vi "FingerMove.vi"() -> ()   [LabVIEW 2013]
uses:
  <vilib>/DAQmx/configure/timing.llb/DAQmx Timing (Implicit).vi
  <vilib>/DAQmx/create/channels.llb/DAQmx Create Channel (CO-Pulse Generation-Frequency).vi
  <vilib>/DAQmx/write.llb/DAQmx Write (Counter Frequency 1Chan 1Samp).vi
  <vilib>/DAQmx/write.llb/DAQmx Write (Digital 1D Bool NChan 1Samp 1Line).vi
  <vilib>/DAQmx/read.llb/DAQmx Read (Counter DBL 1Chan 1Samp).vi
  <vilib>/Platform/TimedLoop/XDataNode/wakeup.ctl
  <vilib>/Platform/TimedLoop/XDataNode/XDNodeRunTimeDep.lvlib
  <vilib>/Platform/TimedLoop/XDataNode/nitl_modes.ctl
  <vilib>/Platform/TimedLoop/XDataNode/timing_clust.ctl
  <vilib>/Platform/TimedLoop/XDataNode/XDataNode.xnode
  <vilib>/addons/Digital Filter Design/NI_DigFilterLicensed.lvlib
  <vilib>/addons/control/pid/NI_PID_pid.lvlib
  <vilib>/DAQmx/write.llb/DAQmx Write (Analog DBL 1Chan 1Samp).vi
  <vilib>/nisyscfg/nisyscfg.lvlib
  SubVIs/VariablesToString_Scalar.vi
  SubVIs/VariablesToString_Array.vi
  <vilib>/addons/control/pid/pid.llb/PID Advanced (DBL Array).vi
  <vilib>/addons/Digital Filter Design/Process.llb/DFD Filtering (PtByPt NChan).vi
  <vilib>/DAQmx/write.llb/DAQmx Write (Analog 1D DBL NChan 1Samp).vi
  SubVIs/VariablesToString_String.vi
  <vilib>/DAQmx/read.llb/DAQmx Read (Analog 1D DBL NChan 1Samp).vi
  <vilib>/addons/Digital Filter Design/_Objects.llb/DFD Filter Structure Type Selector.ctl
  <vilib>/addons/Digital Filter Design/_Objects.llb/DFD Filter Coef.ctl
  <vilib>/addons/Digital Filter Design/_Objects.llb/dfd_Internal Quantization Srcs.ctl
  <vilib>/addons/Digital Filter Design/_Objects.llb/dfd_Internal Quantization Settings.ctl
  <vilib>/addons/Digital Filter Design/_Objects.llb/DFD Coef Norm Type.ctl
  <vilib>/addons/Digital Filter Design/_Objects.llb/DFD Filter Obj.ctl
  <vilib>/Utility/miscctls.llb/LVBoundsTypeDef.ctl
  Control 1.ctl
panel:
  in  "Displacement":dbl[](array[numeric])=[4.95, 5.2, 3.9]
  in  "Middle Reverse Mode":bool
  out "Position, cm":T1(graph)
  out "#SuccessfulBlockTrials":u16
  out "IMT-%Correct":dbl
  out "IMT-Total":dbl
  out "IMT-Success":dbl
  out "MT-%Correct":dbl
  out "MT-Total":dbl
  out "MT-Success":dbl
  out "IT-%Correct":dbl
  out "IT-Total":dbl
  out "IT-Success":dbl
  out "IM-%Correct":dbl
  out "IM-Total":dbl
  out "IM-Success":dbl
  out "Thumb-%Correct":dbl
  out "Thumb-Total":dbl
  out "Thumb-Success":dbl
  out "Middle - %Correct":dbl
  out "Middle - Total":dbl
  out "Middle-Success":dbl
  out "Index-%Correct":dbl
  out "Index-Total":dbl
  out "Index-Success":dbl
  in  "Vis_Center_Y":dbl=0.6
  in  "Vis_Center X":dbl=0.6
  out "#TotalBlockTrials":u16
  in  "Rand_BlockSize":u16=5
  in  "Monkey":string(combo)="Izzle"
  out "GetHostTimeVI":path=path "E:/Code/Tasks/SubVIs/GetHostTime.vi"
  out "AutoCentraVI":path=path "E:/Code/Tasks/SubVIs/AutoCentral.vi"
  out "TaskFolder":path=path "E:/Code/Tasks/FingerMove"
  out "Recording?":bool
  out "CerebusFolder":string="20130418-111956"
  out "StopRecording":bool
  out "Scalefactor":dbl=0.3
  in  "Blank 2":picture
  out "DrawSize 2":T2={"Width"=499, "Height"=304}
  out "Display 2":picture
  out "FingerNum":dbl=1.0
  out "AbortTrials":dbl caption="Total # of Aborts"
  out "FailureTrials":dbl caption="Total # of Failures"
  in  "TrainThresh":dbl[](array[numeric])=[0.5, 0.5, 0.5]
  out "Status":enum16{"In", "Out"}(ring)=enum."Out"
  in  "Radius":dbl=0.44 caption="SuccessRadius"
  in  "MultR":dbl=250.0 caption="DisplayRad"
  out "DrawSize":T2={"Width"=1662, "Height"=1015}
  out "PercentCorrect":dbl caption="Overall - %Correct" format="%#_4g"
  out "SuccessfulTrials":dbl caption="Overall - Successful"
  in  "Pause":bool
  in  "Finger":T3={"Index"=TRUE, "Middle"=FALSE, "Thumb"=FALSE}
  in  "TargetPos":dbl[](array[numeric])=[4.95, 5.2, 3.9]
  in  "Blank":picture
  in  "PIDLimit":dbl=0.5 caption="MaxDutyCycle" min=0.0 max=1.0 step=0.01 format="%.2f"
  out "LP_LoadCell":T4={"mSRate_Fs"=500.0, "mSRate_Version"="2.0", "mSRate_Comments"="", "mSRate_OrgCoef"={"type"=enum."IIR Cascaded Second Order Sections Form II Transposed", "gain"=1.0, "coef a (k)"=[-0.36952737735124136, 0.1958157126558331], "coef b (v)"=[0.20657208382614795, 0.4131441676522959, 0.20657208382614795]}, "mSRate_CurCoef"={"type"=enum."IIR Cascaded Second Order Sections Form II Transposed", "gain"=1.0, "coef a (k)"=[-0.36952737735124136, 0.1958157126558331], "coef b (v)"=[0.20657208382614795, 0.4131441676522959, 0.20657208382614795]}, "mSRate_Quantized?"=FALSE, "mSRate_QCoef"={"type"=enum."Undefined", "gain"=1.0, "coef a (k)"=[], "coef b (v)"=[]}, "mSRate_QSettings"=[], "mSRate_Order"=2, "mSRate_Scaling"={"mSRate_ScaleByPowerOf2?"=FALSE, "mSRate_ScaleType"=enum."No Norm"}} {"mSRate_QSettings"."source" items=["Coef a/k"=0, "Coef b/v"=7, "Input"=1, "Output"=2, "Multiplicand"=3, "Product"=4, "Sum"=5, "Delay"=6, "Gain"=8]}
  out "PWMTaskA":refnum<k21>
  out "PIDSlowLoop":bool
  out "PIDLoopTime(us)":i64=881 caption="Actual Loop Period (us)"
  out "PIDLoopPeriod(s)":dbl=0.002 caption="Loop Period PID (s)" format="%#_10g"
  out "PWMTaskB":refnum<k21>
  in  "Stop":bool
  out "SetPoint":dbl[](array[numeric])=[1.0, 2.0, 1.0] caption="Set Point" min=-10.0 max=10.0 step=1.0
  in  "PIDLoopFreq(Hz)":dbl=500.0 caption="Loop Period (us)"
  out "PWMTaskC":refnum<k21>
  out "MotorDir":bool[](array[boolean])=[TRUE, TRUE, TRUE]
  in  "LP_LoadCell(Hz)":dbl=100.0
  in  "BndrsCluster":T10={"InwardLimit(%)"=[0.75, 0.8, 0.6], "OutwardLimit(%)"=[0.25, 0.2, 0.4], "SpringCnst"=[5.0, 5.0, 5.0]} caption="Boundaries"
  out "EncMax":dbl[](array[numeric])
  in  "PWMFreq(Hz)":dbl=20000.0 caption="PWM (Hz)" format="%#.6f"
  in  "PIDGains":T11={"proportional high (Kc)"=0.2, "integral high (Ti, min)"=0.0, "derivative high (Td, min)"=0.0, "derivative low (Td, min)"=0.0, "integral low (Ti, min)"=0.0, "proportional low (Kc)"=0.1} caption="PID Gains"
  out "PIDGainsOut":T12(array[cluster])=[{"proportional gain (Kc)"=0.4600000000000001, "integral time (Ti, min)"=0.0, "derivative time (Td, min)"=0.0}, {"proportional gain (Kc)"=0.42000000000000004, "integral time (Ti, min)"=0.0, "derivative time (Td, min)"=0.0}, {"proportional gain (Kc)"=0.4600000000000001, "integral time (Ti, min)"=0.0, "derivative time (Td, min)"=0.0}]
  in  "Linearity":dbl=1.0 format="%.2f"
  out "Outcome":string="--"
  out "Current State":T13(ring)=enum."Acquire Start"
  out "Finalize":enum16{"Reward", "Cerebus", "Reset"}(ring)
  out "LoopCount":u64=13080
  out "TrialCount":i32=1 caption="Overall - Total Trials"
  out "EncPos":cluster{"[0]":dbl, "[1]":dbl, "[2]":dbl}(graph) caption="Position"
  in  "InitialPos":dbl[](array[numeric])=[4.95, 5.2, 3.9]
  out "LoadCell":cluster{"[0]":dbl, "[1]":dbl, "[2]":dbl}(graph)={"[0]"=0.5361853302770733, "[1]"=0.5356007172382269, "[2]"=0.5346289515190896} caption="Force, lbs"
  out "SetPtOut":cluster{"[0]":dbl, "[1]":dbl, "[2]":dbl}(graph)={"[0]"=1.0, "[1]"=2.0, "[2]"=1.0} caption="Set Point, lbs"
  in  "InitialForce":dbl[](array[numeric])=[1.0, 2.0, 1.0] min=-10.0 max=10.0 step=1.0
  in  "RandFinger":bool
  out "StartTime":timestamp=timestamp(3449121258.124381 s since 1904-01-01)
  out "TaskType":string="FingerMove.vi"
  out "DatabaseUDL":path=path "E:/Data/Setup2Database.udl"
  in  "RecordsSelection":string(combo)
  in  "Database":T14={"ExperimentDate"=timestamp(3449121258.124381 s since 1904-01-01), "ImplantDate"=timestamp(3449023200 s since 1904-01-01), "CerebusFolder"="20130418-111956", "Experimenter"="Cody Barton", "NHPName"="Frak", "DeviceType"="USEA", "DeviceSerial"="CG-64BPX-F419", "DeviceHemisphere"="right", "DeviceRegion"="median nerve", "TaskType"="FingerMove.vi", "TaskComments"="test123", "RecordingComments"="test123", "GeneralObservations"="test123"}
  in  "CerebusConfigFile":path=path "E:/Code/Tasks/FingerMove/CerebusConfigBehavior20130507.mat"
  in  "Timing":T15={"JuiceTime"=1700.0, "AbortTime"=2000.0, "ARD"=1500.0, "HoldTime"=500.0, "ASD"=1000.0}
  out "Display":picture
  out "LoopPeriod":u64=10
  out "SlowLoop":bool
  out "LoopTime":i64=381
  # "Do not place ';' or '=' in the comment fields"
  # "all time in ms"
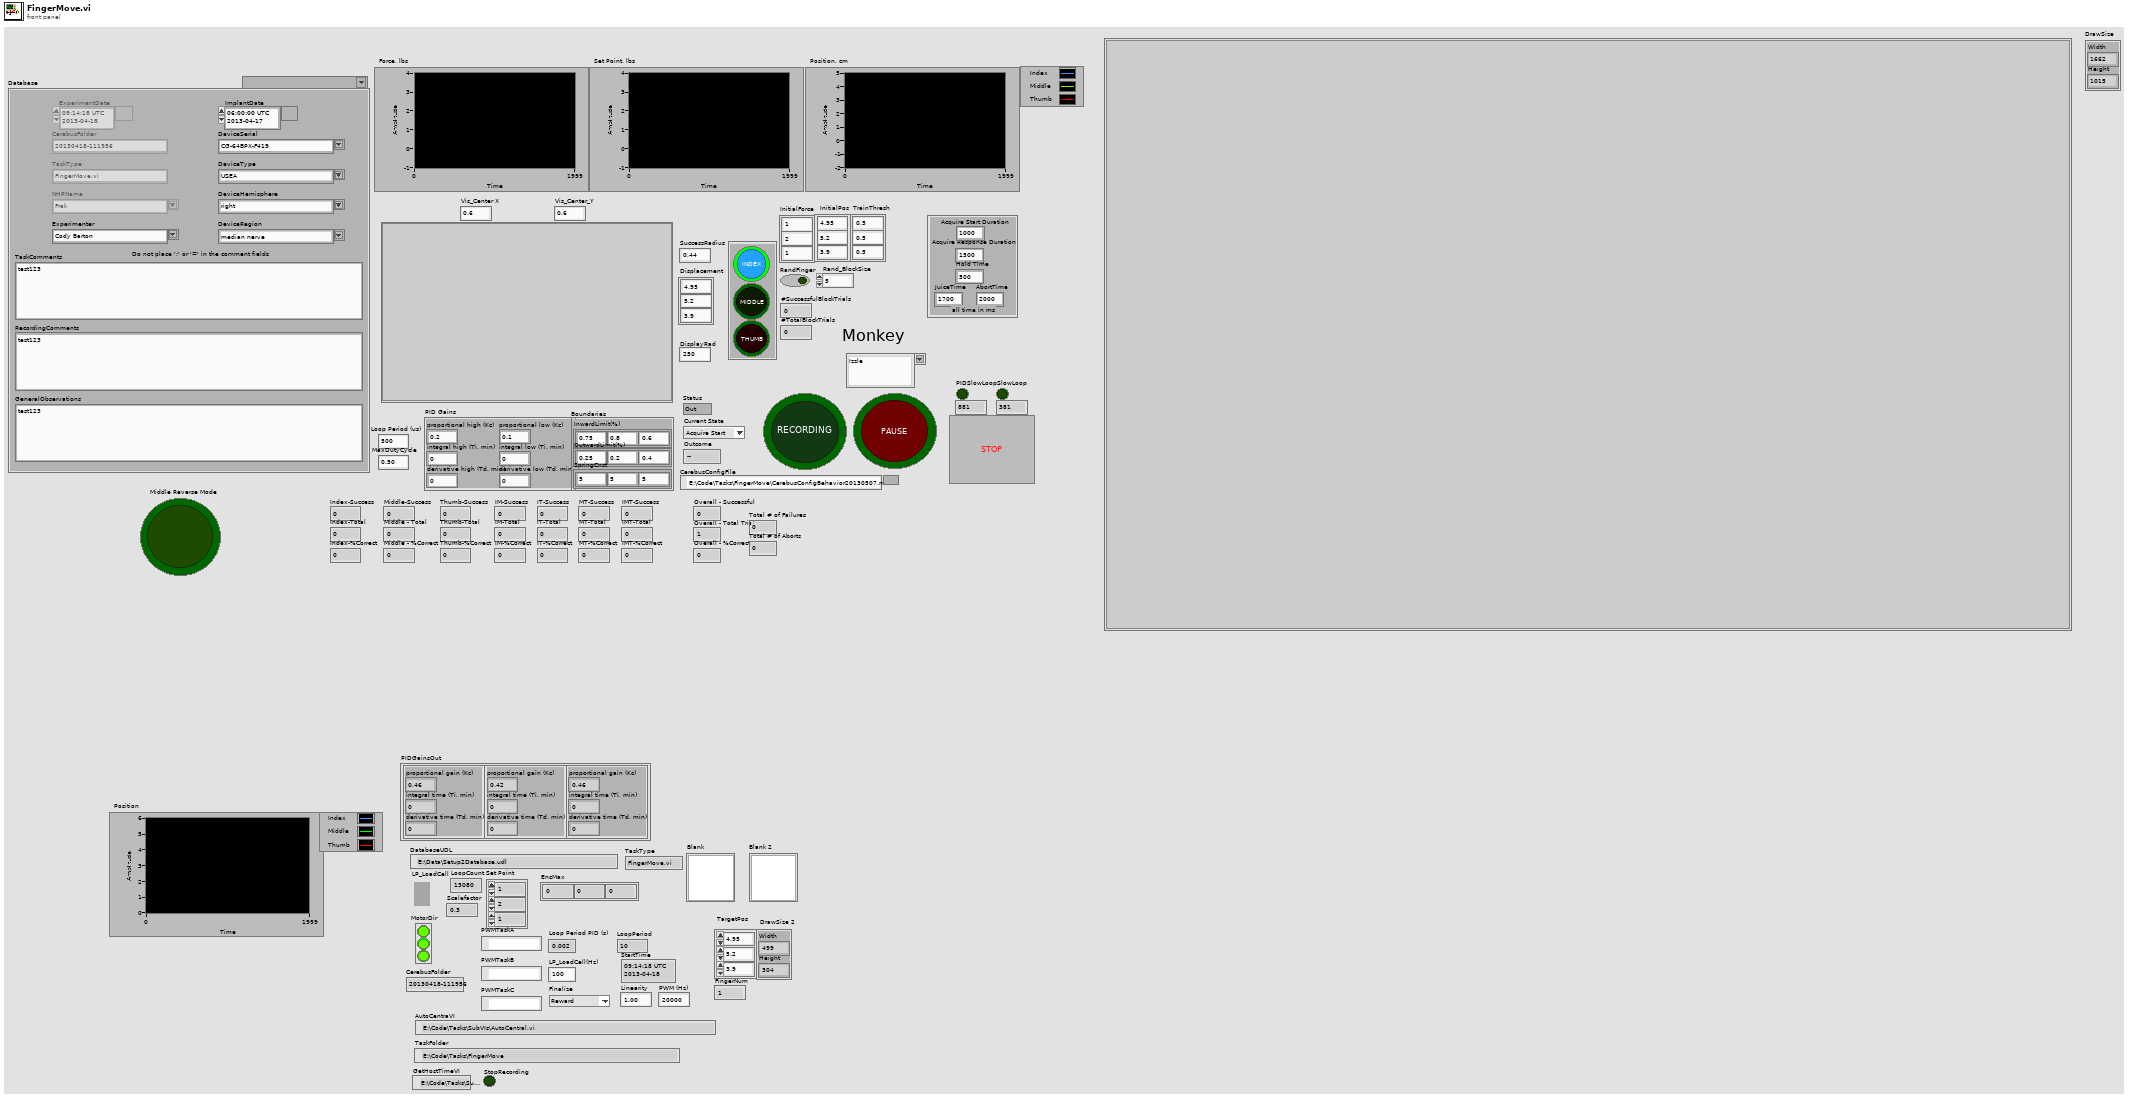
[diagram p1: front panel]
types:
  T1 = cluster{"[0]":dbl, "[1]":dbl, "[2]":dbl, "[3]":dbl, "[4]":dbl, "[5]":dbl, "[6]":dbl, "[7]":dbl, "[8]":dbl}
  T2 = typedef "LVBoundsTypeDef.ctl" = cluster{"Width":u32, "Height":u32}
  T3 = cluster{"Index":bool, "Middle":bool, "Thumb":bool}
  T4 = typedef "NI_DigFilterLicensed.lvlib/DFD Filter Obj.ctl" = cluster{"mSRate_Fs":dbl, "mSRate_Version":string, "mSRate_Comments":string, "mSRate_OrgCoef":T5, "mSRate_CurCoef":T5, "mSRate_Quantized?":bool, "mSRate_QCoef":T5, "mSRate_QSettings":T7[], "mSRate_Order":i32, "mSRate_Scaling":cluster{"mSRate_ScaleByPowerOf2?":bool, "mSRate_ScaleType":T9}}
  T5 = typedef "NI_DigFilterLicensed.lvlib/DFD Filter Coef.ctl" = cluster{"type":T6, "gain":dbl, "coef a (k)":dbl[], "coef b (v)":dbl[]}
  T6 = typedef "NI_DigFilterLicensed.lvlib/DFD Filter Structure Type Selector.ctl" = enum16{"Undefined", "FIR Direct Form", "FIR Direct Form Transposed", "FIR Symmetric", "FIR Antisymmetric", "IIR Direct Form I", "IIR Direct Form I Transposed", "IIR Direct Form II", "IIR Direct Form II Transposed", "IIR Cascaded Second Order Sections Form I", "IIR Cascaded Second Order Sections Form I Transposed", "IIR Cascaded Second Order Sections Form II", "IIR Cascaded Second Order Sections Form II Transposed", "Lattice Allpass (basic sections)", "Lattice Allpass (one multiplier sections)", "Lattice Allpass (normalized sections)", "Lattice AR (basic sections)", "Lattice AR (one multiplier sections)", "Lattice AR (normalized sections)", "Lattice MA (minimum phase)", "Lattice MA (maximum phase)", "Lattice ARMA (basic sections)", "Lattice ARMA (one multiplier sections)", "Lattice ARMA (normalized sections)"}
  T7 = typedef "NI_DigFilterLicensed.lvlib/dfd_Internal Quantization Settings.ctl" = cluster{"source":T8, "wl":i16, "iwl":i16, "overflow mode":enum16{"Saturation", "Wrap"}, "rounding mode":enum16{"Nearest", "Truncation"}, "signed?":bool}
  T8 = typedef "NI_DigFilterLicensed.lvlib/dfd_Internal Quantization Srcs.ctl" = u16
  T9 = typedef "NI_DigFilterLicensed.lvlib/DFD Coef Norm Type.ctl" = enum16{"No Norm", "Time Domain 1-Norm", "Time Domain 2-Norm", "Time Domain Inf-Norm"}
  T10 = cluster{"InwardLimit(%)":dbl[], "OutwardLimit(%)":dbl[], "SpringCnst":dbl[]}
  T11 = cluster{"proportional high (Kc)":dbl, "integral high (Ti, min)":dbl, "derivative high (Td, min)":dbl, "derivative low (Td, min)":dbl, "integral low (Ti, min)":dbl, "proportional low (Kc)":dbl}
  T12 = cluster{"proportional gain (Kc)":dbl, "integral time (Ti, min)":dbl, "derivative time (Td, min)":dbl}[]
  T13 = enum16{"Initialize", "Acquire Start", "Acquire Response", "Finalize"}
  T14 = cluster{"ExperimentDate":timestamp, "ImplantDate":timestamp, "CerebusFolder":string, "Experimenter":string, "NHPName":string, "DeviceType":string, "DeviceSerial":string, "DeviceHemisphere":string, "DeviceRegion":string, "TaskType":string, "TaskComments":string, "RecordingComments":string, "GeneralObservations":string}
  T15 = typedef "Control 1.ctl" = cluster{"JuiceTime":dbl, "AbortTime":dbl, "ARD":dbl, "HoldTime":dbl, "ASD":dbl}
  T16 = enum16{"Initialize", "String", "Start", "New Session", "Stop", "Resume", "Close"}
  T17 = cluster{"JuiceTime":dbl, "AbortTime":dbl, "ARD":dbl, "HoldTime":dbl, "ASD":dbl}
  T18 = cluster{"ExperimentDate":timestamp, "ImplantDate":timestamp, "CerebusFolder":string, "Experimenter":string, "NHP Name":string, "DeviceType":string, "DeviceSerial":string, "DeviceHemisphere":string, "DeviceRegion":string, "TaskType":string, "TaskComments":string, "RecordingComments":string, "GeneralObservations":string}
  T19 = enum16{"SaveConfiguration", "StartRecording", "StopRecording"}
  T20 = typedef "XDNodeRunTimeDep.lvlib/timing_clust.ctl" = cluster{"Expected End [f-1]":u64, "Actual End [f-1]":u64, "Finished Late? [f-1]":bool, "Expected End [i-1]":u64, "Actual End [i-1]":u64, "Finished Late? [i-1]":bool, "Expected Start [i]":u64, "Actual Start [i]":u64, "Expected Start [f]":u64, "Actual Start [f]":u64, "Source Name":string, "Structure Name":string, "Period":i64, "Deadline":i64, "Offset":i64, "Start":i64, "Priority":i32, "Timeout":i32, "Mode":T21, "Wakeup Reason":T22, "Error":errorcluster, "Source Type":string, "Secondary Source Type":string, "Global End Time":u64, "Global Start Time":u64, "Frame Duration":u64, "Iteration Duration":u64, "Assigned CPU":i32, "I/O Scan Engine Mode":u32}
  T21 = typedef "XDNodeRunTimeDep.lvlib/nitl_modes.ctl" = enum32{"No Change", "Process missed periods, maintain original phase", "Discard missed periods, maintain original phase", "Process missed periods, ignore original phase", "Discard missed periods, ignore original phase"}
  T22 = typedef "XDNodeRunTimeDep.lvlib/wakeup.ctl" = enum32{"Normal", "Aborted", "Asynchronous wakeup", "Timing source error", "Timed loop error", "Timeout"}
  T23 = enum16{"Lowpass", "Highpass", "Bandpass", "Bandstop"}
  T24 = cluster{"left":i16, "left":i16, "Width":u32, "Height":u32}
  T25 = cluster{"SetPointOut[0]":dbl, "SetPointOut[1]":dbl, "SetPointOut[2]":dbl}
  T26 = cluster{"signal out[0]":dbl, "signal out[1]":dbl, "signal out[2]":dbl}
  T27 = typedef "LVAllMonitorsDisplayTypeDef.ctl" = cluster{"Bounds":cluster{"Left":i16, "Top":i16, "Right":i16, "Bottom":i16}, "Depth":i16}[]
  T28 = cluster{"Disp.AllMonitors[0]":cluster{"Bounds":cluster{"Left":i16, "Top":i16, "Right":i16, "Bottom":i16}, "Depth":i16}, "Disp.AllMonitors[1]":cluster{"Bounds":cluster{"Left":i16, "Top":i16, "Right":i16, "Bottom":i16}, "Depth":i16}, "Disp.AllMonitors[2]":cluster{"Bounds":cluster{"Left":i16, "Top":i16, "Right":i16, "Bottom":i16}, "Depth":i16}, "Disp.AllMonitors[3]":cluster{"Bounds":cluster{"Left":i16, "Top":i16, "Right":i16, "Bottom":i16}, "Depth":i16}, "Disp.AllMonitors[4]":cluster{"Bounds":cluster{"Left":i16, "Top":i16, "Right":i16, "Bottom":i16}, "Depth":i16}, "Disp.AllMonitors[5]":cluster{"Bounds":cluster{"Left":i16, "Top":i16, "Right":i16, "Bottom":i16}, "Depth":i16}, "Disp.AllMonitors[6]":cluster{"Bounds":cluster{"Left":i16, "Top":i16, "Right":i16, "Bottom":i16}, "Depth":i16}, "Disp.AllMonitors[7]":cluster{"Bounds":cluster{"Left":i16, "Top":i16, "Right":i16, "Bottom":i16}, "Depth":i16}, "Disp.AllMonitors[8]":cluster{"Bounds":cluster{"Left":i16, "Top":i16, "Right":i16, "Bottom":i16}, "Depth":i16}}
  T29 = typedef "LVRectTypeDef.ctl" = cluster{"Left":i16, "Top":i16, "Right":i16, "Bottom":i16}
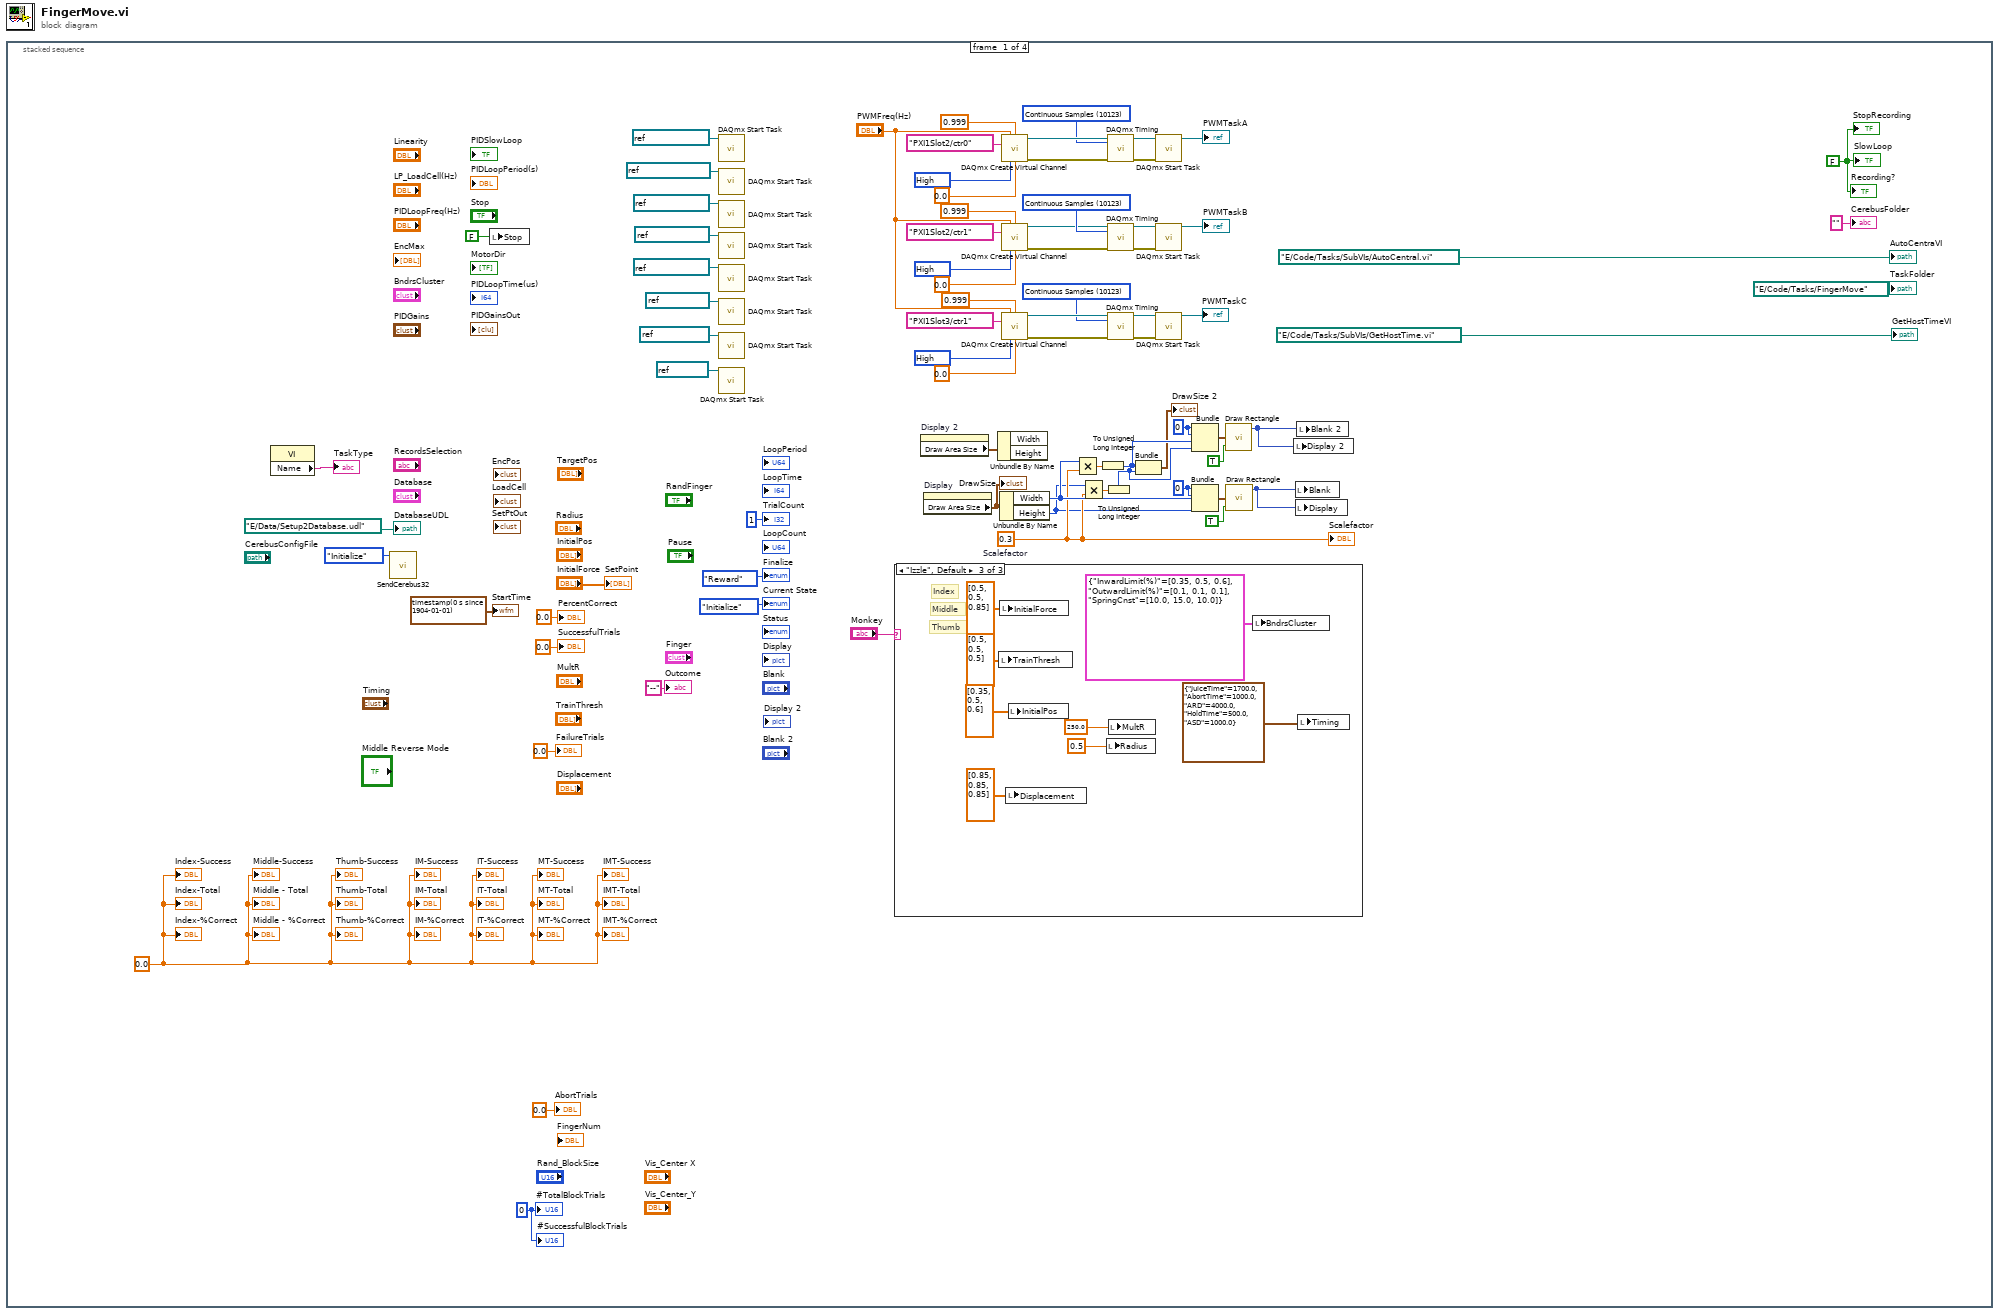
[diagram p0: block diagram]
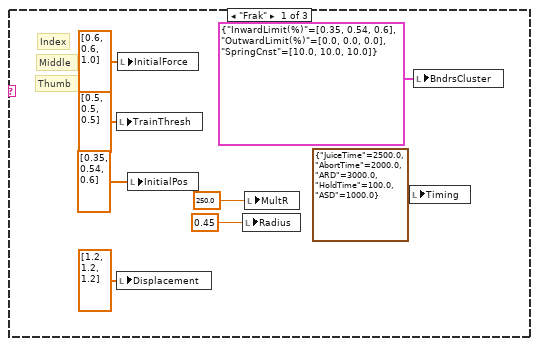
[diagram p2: hidden frame]
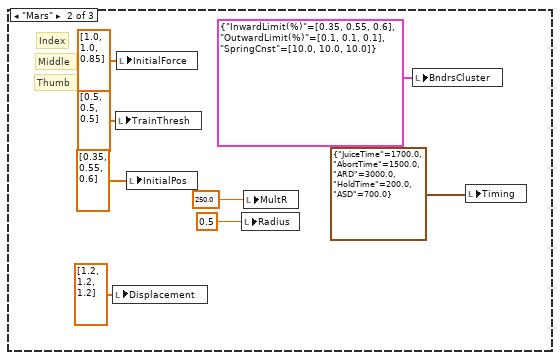
[diagram p3: hidden frame]
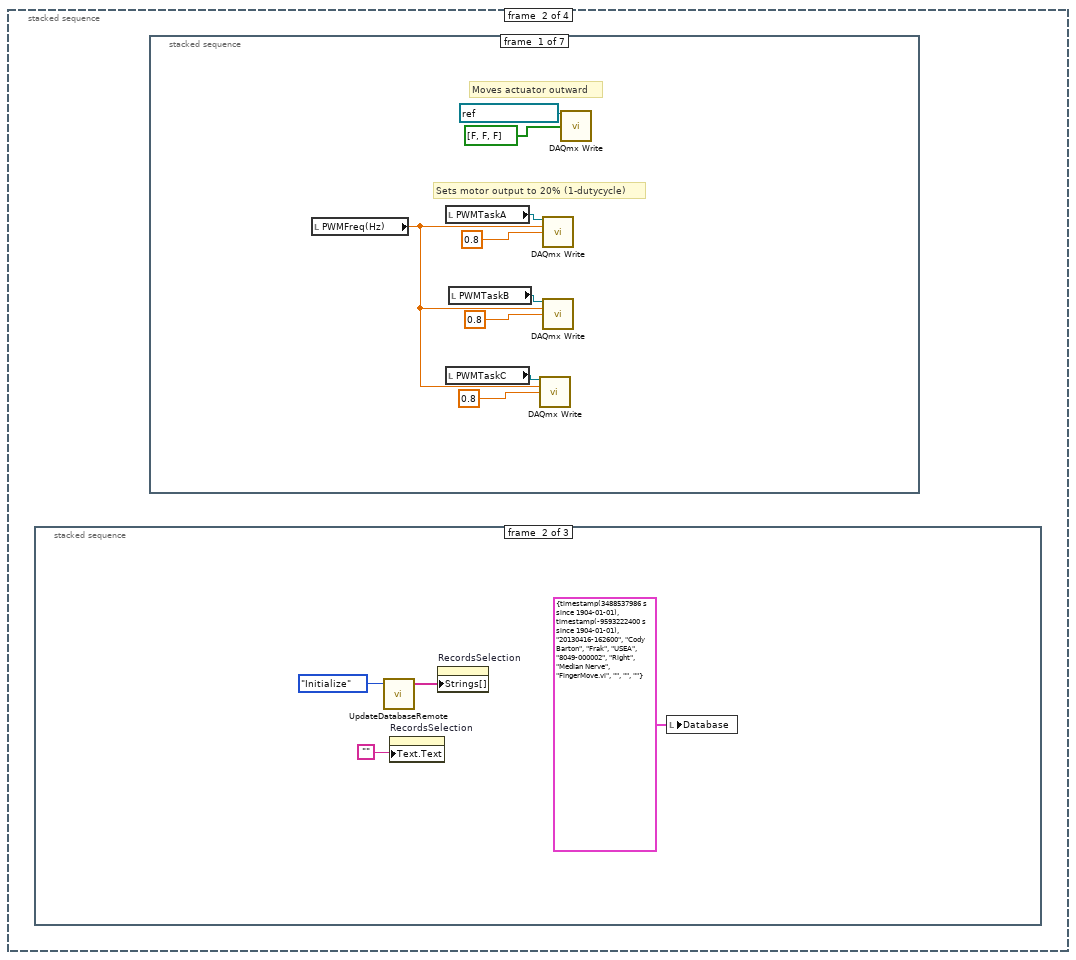
[diagram p4: hidden frame]
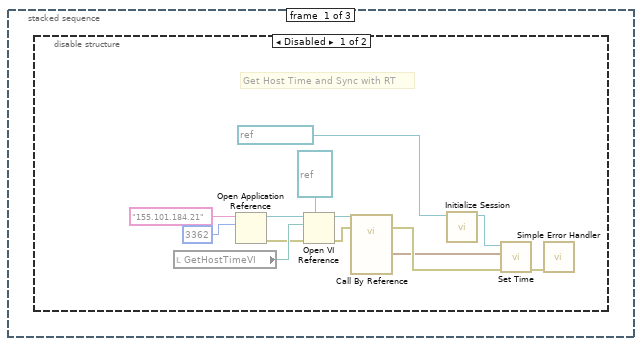
[diagram p5: hidden frame]
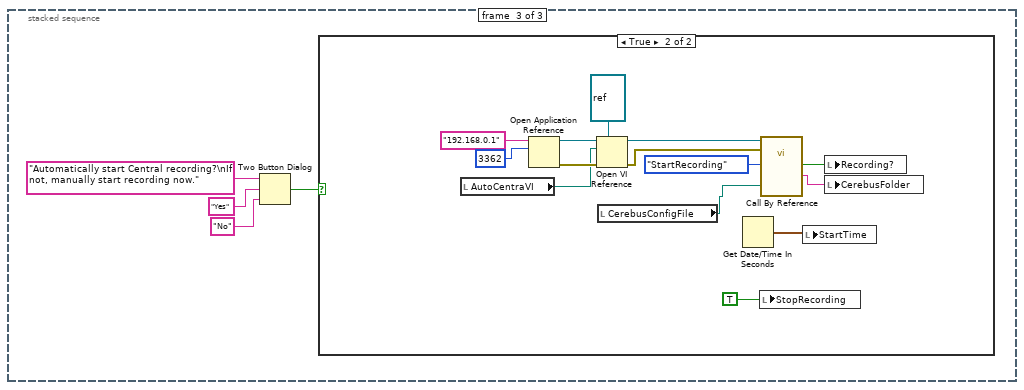
[diagram p7: hidden frame]
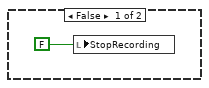
[diagram p8: hidden frame]
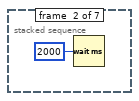
[diagram p9: hidden frame]
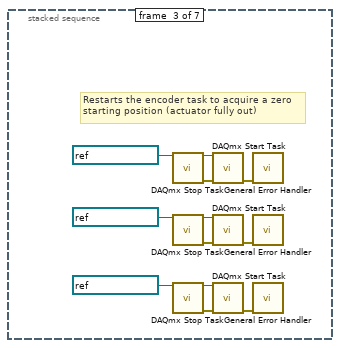
[diagram p10: hidden frame]
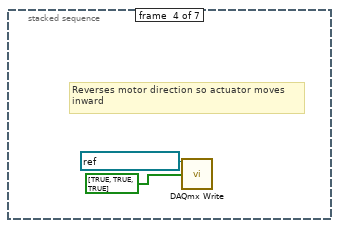
[diagram p11: hidden frame]
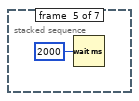
[diagram p12: hidden frame]
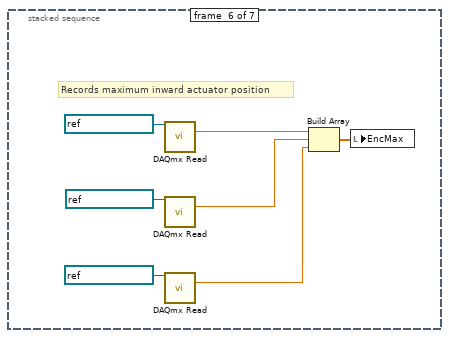
[diagram p13: hidden frame]
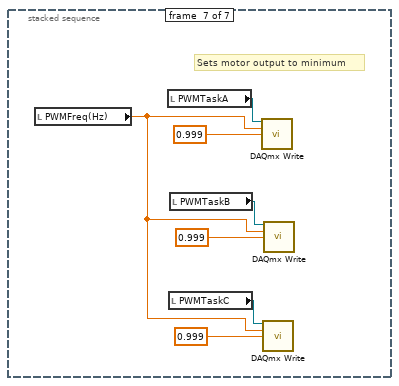
[diagram p14: hidden frame]
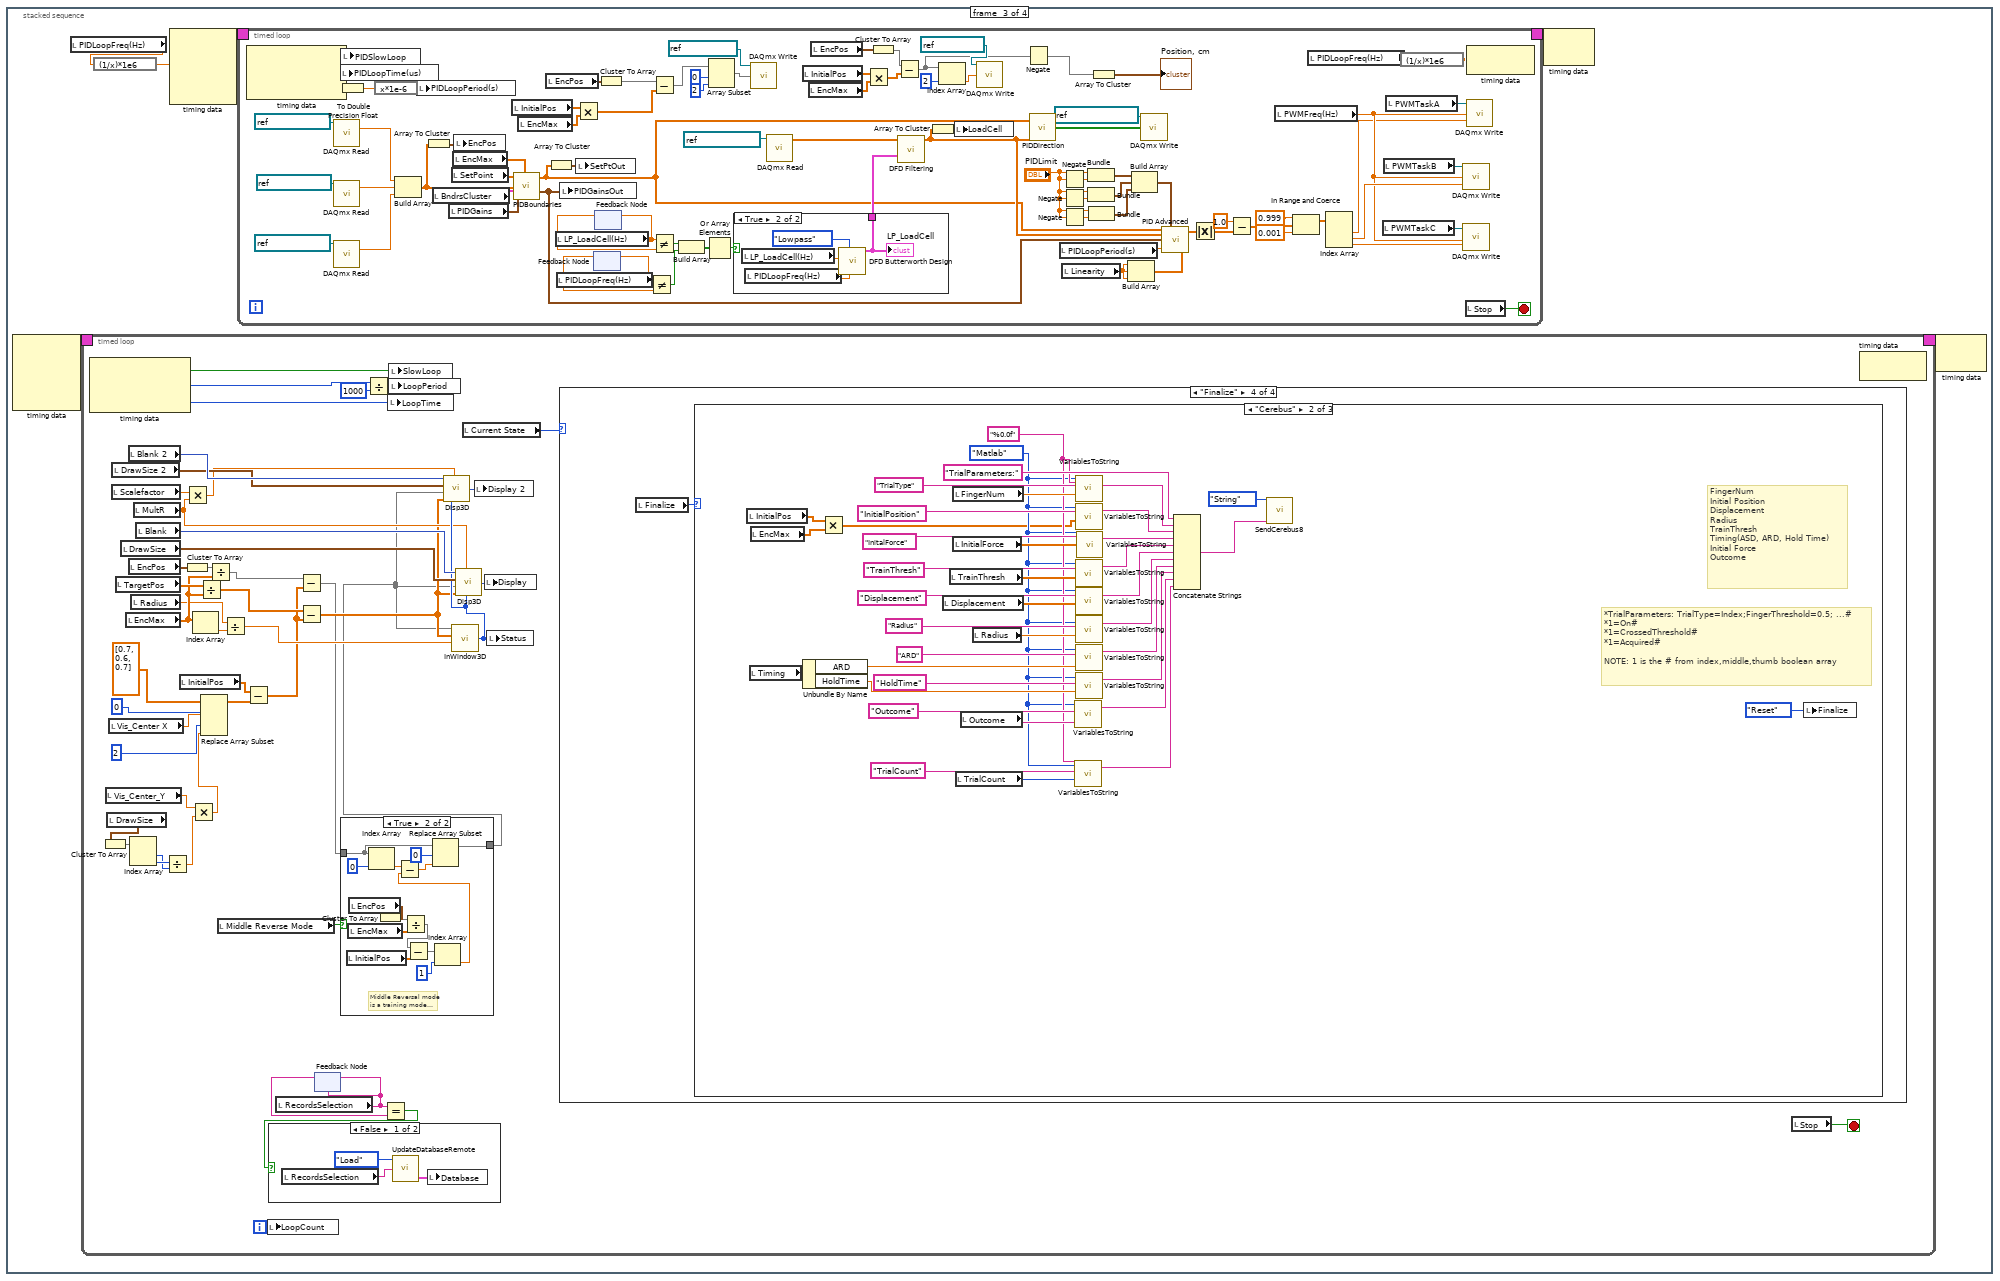
[diagram p15: hidden frame]
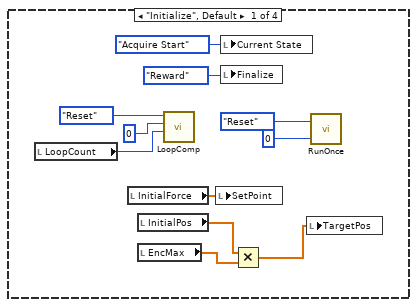
[diagram p18: hidden frame]
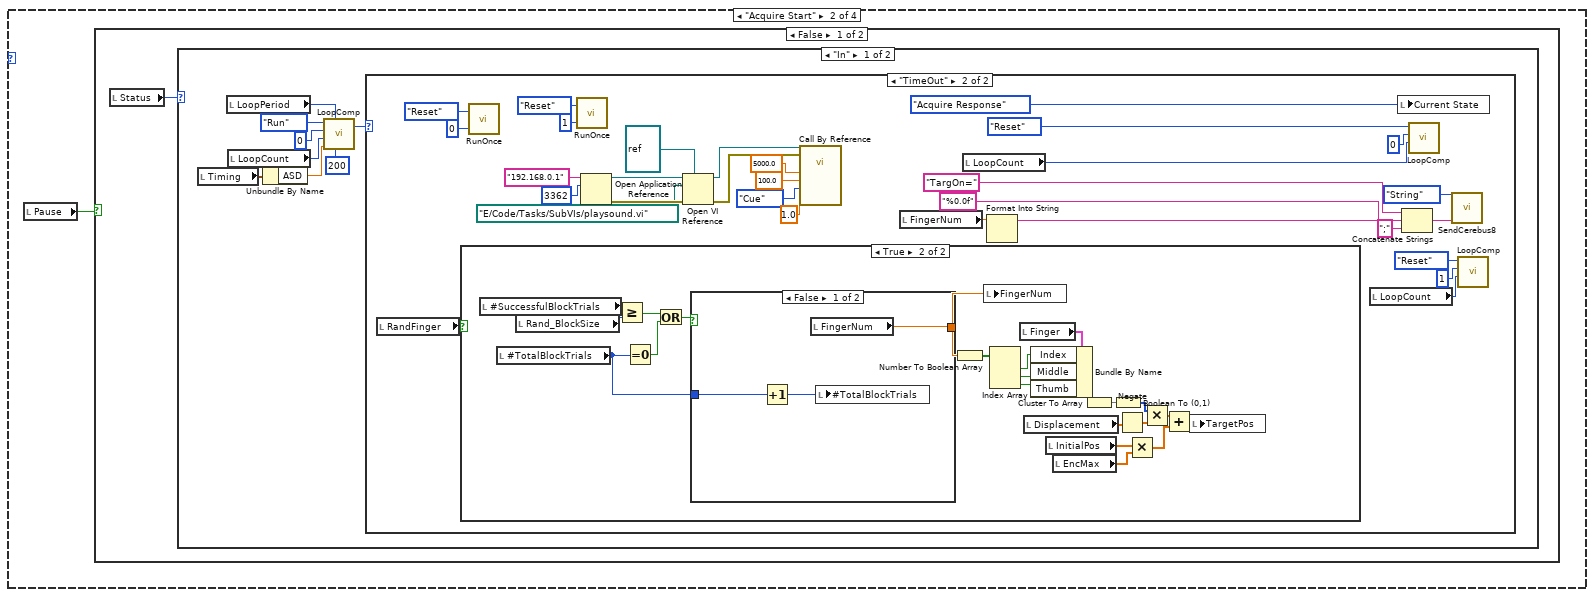
[diagram p19: hidden frame]
diagram:
  n1 = stacked-sequence {
    frame #0 {
      w2 = 0.0
      w1 = 0
      w3 = FALSE ("StopRecording")
      w21 = 0.3  # Scalefactor
      w25 = i16 0 ("left")
      w29 = i16 0 ("left")
      w52 = 10192 items=["High"=10192, "Low"=10214] ("idle state")
      w46 = 10123 items=["Finite Samples"=10178, "Continuous Samples"=10123] ("sample mode")
      w59 = 10192 items=["High"=10192, "Low"=10214] ("idle state")
      w65 = 10123 items=["Finite Samples"=10178, "Continuous Samples"=10123] ("sample mode")
      w76 = 10192 items=["High"=10192, "Low"=10214] ("idle state")
      w69 = 10123 items=["Finite Samples"=10178, "Continuous Samples"=10123] ("sample mode")
      n2 = property class="VI"() -> ("Name"=→"TaskType":string)  [unwired: 2 in, 2 out]
      n3 = call "SendCerebus32.vi"("Mode"=T16."Initialize") -> ()  [unwired: 4 in]
      n4 = local write "Stop"(FALSE ("stop")) -> ()
      n5 = call <vilib>:"DAQmx Start Task.vi"("task/channels in"=refnum<k21> "ForceInABC") -> ()  [unwired: 13 in, 2 out]
      n6 = call <vilib>:"DAQmx Start Task.vi"("task/channels in"=refnum<k21> "MotorDirABC") -> ()  [unwired: 13 in, 2 out]
      n7 = call <vilib>:"DAQmx Start Task.vi"("task/channels in"=refnum<k21> "PositionInA") -> ()  [unwired: 13 in, 2 out]
      n8 = call <vilib>:"DAQmx Start Task.vi"("task/channels in"=refnum<k21> "PositionInB" ("task")) -> ()  [unwired: 13 in, 2 out]
      n9 = call <vilib>:"DAQmx Start Task.vi"("task/channels in"=refnum<k21> "PositionInC") -> ()  [unwired: 13 in, 2 out]
      n10 = call <vilib>:"DAQmx Start Task.vi"("task/channels in"=refnum<k21> "PosOutT" ("task")) -> ()  [unwired: 13 in, 2 out]
      n11 = call <vilib>:"DAQmx Start Task.vi"("task/channels in"=refnum<k21> "PosOutIM") -> ()  [unwired: 13 in, 2 out]
      n12 = call <vilib>:"DAQmx Start Task.vi"("task/channels in"=refnum<k21> "sound") -> ()  [unwired: 13 in, 2 out]
      n13 = case shown="\"Izzle\", Default" "Monkey" {
        frame "Frak" {
          # "Thumb"
          # "Middle"
          # "Index"
          n14 = local write "TrainThresh"(dbl[] [0.5, 0.5, 0.5] ("InitialForce")) -> ()
          n15 = local write "Displacement"(dbl[] [1.2, 1.2, 1.2] ("InitialPos")) -> ()
          n16 = local write "InitialForce"(dbl[] [0.6, 0.6, 1.0] ("InitialForce")) -> ()
          n17 = local write "InitialPos"(dbl[] [0.35, 0.54, 0.6] ("InitialPos")) -> ()
          n18 = local write "Radius"(0.45 ("Displacement")) -> ()
          n19 = local write "MultR"(250.0 ("Displacement")) -> ()
          n20 = local write "Timing"(T17 {"JuiceTime"=2500.0, "AbortTime"=2000.0, "ARD"=3000.0, "HoldTime"=100.0, "ASD"=1000.0} ("Timing")) -> ()
          n21 = local write "BndrsCluster"(T10 {"InwardLimit(%)"=[0.35, 0.54, 0.6], "OutwardLimit(%)"=[0.0, 0.0, 0.0], "SpringCnst"=[10.0, 10.0, 10.0]} ("BndrsCluster")) -> ()
        }
        frame "Mars" {
          # "Thumb"
          # "Middle"
          # "Index"
          n22 = local write "Displacement"(dbl[] [1.2, 1.2, 1.2] ("InitialPos")) -> ()
          n23 = local write "TrainThresh"(dbl[] [0.5, 0.5, 0.5] ("InitialForce")) -> ()
          n24 = local write "InitialForce"(dbl[] [1.0, 1.0, 0.85] ("InitialForce")) -> ()
          n25 = local write "InitialPos"(dbl[] [0.35, 0.55, 0.6] ("InitialPos")) -> ()
          n26 = local write "Radius"(0.5 ("Displacement")) -> ()
          n27 = local write "MultR"(250.0 ("Displacement")) -> ()
          n28 = local write "BndrsCluster"(T10 {"InwardLimit(%)"=[0.35, 0.55, 0.6], "OutwardLimit(%)"=[0.1, 0.1, 0.1], "SpringCnst"=[10.0, 10.0, 10.0]} ("BndrsCluster")) -> ()
          n29 = local write "Timing"(T17 {"JuiceTime"=1700.0, "AbortTime"=1500.0, "ARD"=3000.0, "HoldTime"=200.0, "ASD"=700.0} ("Timing")) -> ()
        }
        frame "Izzle", Default {
          # "Thumb"
          # "Middle"
          # "Index"
          n30 = local write "TrainThresh"(dbl[] [0.5, 0.5, 0.5] ("InitialForce")) -> ()
          n31 = local write "InitialForce"(dbl[] [0.5, 0.5, 0.85] ("InitialForce")) -> ()
          n32 = local write "Displacement"(dbl[] [0.85, 0.85, 0.85] ("InitialForce")) -> ()
          n33 = local write "InitialPos"(dbl[] [0.35, 0.5, 0.6] ("InitialPos")) -> ()
          n34 = local write "Radius"(0.5 ("Displacement")) -> ()
          n35 = local write "MultR"(250.0 ("Displacement")) -> ()
          n36 = local write "BndrsCluster"(T10 {"InwardLimit(%)"=[0.35, 0.5, 0.6], "OutwardLimit(%)"=[0.1, 0.1, 0.1], "SpringCnst"=[10.0, 15.0, 10.0]} ("BndrsCluster")) -> ()
          n37 = local write "Timing"(T17 {"JuiceTime"=1700.0, "AbortTime"=1000.0, "ARD"=4000.0, "HoldTime"=500.0, "ASD"=1000.0} ("Timing")) -> ()
        }
      }
      n38 = property on="Display 2" class="Pict"() -> ("Draw Area Size"=w24:T2)  [unwired: 2 in, 2 out]
      n39 = property on="Display" class="Pict"() -> ("Draw Area Size"=w28:T2)  [unwired: 2 in, 2 out]
      "DrawSize" <- w28
      n40 = Unbundle By Name(w24) -> ()  [unwired: 2 out]
      n41 = Unbundle By Name(w28) -> ("Width"=w23:u32, "Height"=w20:u32)
      n42 = call-poly <vilib>:"DAQmx Create Virtual Channel.vi"("frequency"="PWMFreq(Hz)", "duty cycle"=0.999, "counter"=tag "PXI1Slot2/ctr0", "idle state"=w76, "initial delay"=0.0) -> ("task out"=w72:refnum<k21>, "error out"=w73:errorcluster)  [unwired: 9 in]
      n43 = call-poly <vilib>:"DAQmx Create Virtual Channel.vi"("frequency"="PWMFreq(Hz)", "duty cycle"=0.999, "counter"=tag "PXI1Slot2/ctr1", "idle state"=w59, "initial delay"=0.0) -> ("task out"=w62:refnum<k21>, "error out"=w61:errorcluster)  [unwired: 9 in]
      n44 = call-poly <vilib>:"DAQmx Create Virtual Channel.vi"("frequency"="PWMFreq(Hz)", "duty cycle"=0.999, "counter"=tag "PXI1Slot3/ctr1", "idle state"=w52, "initial delay"=0.0) -> ("task out"=w49:refnum<k21>, "error out"=w50:errorcluster)  [unwired: 9 in]
      n45 = Multiply(x=w23, y=w21) -> (x*y=w22:dbl)
      n46 = Multiply(x=w20, y=w21) -> (x*y=w19:dbl)
      n47 = To Unsigned Long Integer(number=w22) -> (unsigned 32bit integer=w18:u32)
      n48 = To Unsigned Long Integer(number=w19) -> (unsigned 32bit integer=w17:u32)
      n49 = call-poly <vilib>:"DAQmx Timing.vi"("task/channels in"=w72, "sample mode"=w69, "error in"=w73) -> ("task out"=w70:refnum<k21>, "error out"=w71:errorcluster)  [unwired: 11 in]
      n50 = call-poly <vilib>:"DAQmx Timing.vi"("task/channels in"=w62, "sample mode"=w65, "error in"=w61) -> ("task out"=w64:refnum<k21>, "error out"=w63:errorcluster)  [unwired: 11 in]
      n51 = call-poly <vilib>:"DAQmx Timing.vi"("task/channels in"=w49, "sample mode"=w46, "error in"=w50) -> ("task out"=w47:refnum<k21>, "error out"=w48:errorcluster)  [unwired: 11 in]
      n52 = Bundle(w18, w17) -> (→"DrawSize 2":cluster{u32, u32})  [unwired: 1 in]
      n53 = call <vilib>:"DAQmx Start Task.vi"("task/channels in"=w70, "error in"=w71) -> ("task out"=→"PWMTaskA":refnum<k21>)  [unwired: 12 in, 1 out]
      n54 = call <vilib>:"DAQmx Start Task.vi"("task/channels in"=w64, "error in"=w63) -> ("task out"=→"PWMTaskB":refnum<k21>)  [unwired: 12 in, 1 out]
      n55 = call <vilib>:"DAQmx Start Task.vi"("task/channels in"=w47, "error in"=w48) -> ("task out"=→"PWMTaskC":refnum<k21>)  [unwired: 12 in, 1 out]
      n56 = Bundle("left"=w25, "left"=w25, w18, w17) -> (w12:cluster{"left":i16, "left":i16, u32, u32})  [unwired: 1 in]
      n57 = Bundle("left"=w29, "left"=w29, "Width"=w23, "Height"=w20) -> (w13:T24)  [unwired: 1 in]
      n58 = call <vilib>:"Draw Rectangle.vi"("rect"=w12, "fill?(F)"=TRUE) -> ("new picture"=w10:picture)  [unwired: 7 in]
      n59 = call <vilib>:"Draw Rectangle.vi"("rect"=w13, "fill?(F)"=TRUE) -> ("new picture"=w14:picture)  [unwired: 7 in]
      n60 = local write "Display 2"(w10) -> ()
      n61 = local write "Blank"(w14) -> ()
      n62 = local write "Display"(w14) -> ()
      n63 = local write "Blank 2"(w10) -> ()
      "SetPoint" <- "InitialForce"
      "Outcome" <- "--" ("Outcome")
      "Current State" <- T13."Initialize" ("Current State")
      "Finalize" <- enum16{"Reward", "Cerebus", "Reset"}."Reward" ("Finalize")
      "TrialCount" <- 1 ("TrialCount")
      "StartTime" <- timestamp(0 s since 1904-01-01)
      "DatabaseUDL" <- path "E:/Data/Setup2Database.udl" ("DatabaseUDL")
      "SlowLoop" <- w3
      "PercentCorrect" <- 0.0 ("PercentCorrect")
      "SuccessfulTrials" <- 0.0 ("SuccessfulTrials")
      "FailureTrials" <- 0.0 ("FailureTrials")
      "AbortTrials" <- 0.0 ("AbortTrials")
      "Scalefactor" <- w21
      "StopRecording" <- w3
      "CerebusFolder" <- "" ("CerebusFolder")
      "Recording?" <- w3
      "AutoCentraVI" <- path "E:/Code/Tasks/SubVIs/AutoCentral.vi" ("AutoCentraVI")
      "TaskFolder" <- path "E:/Code/Tasks/FingerMove" ("SaccadeFolder")
      "GetHostTimeVI" <- path "E:/Code/Tasks/SubVIs/GetHostTime.vi" ("GetHostTimeVI")
      "#TotalBlockTrials" <- w1
      "Index-Success" <- w2
      "Index-Total" <- w2
      "Index-%Correct" <- w2
      "Middle-Success" <- w2
      "Middle - Total" <- w2
      "Middle - %Correct" <- w2
      "Thumb-Success" <- w2
      "Thumb-Total" <- w2
      "Thumb-%Correct" <- w2
      "IM-Success" <- w2
      "IM-Total" <- w2
      "IM-%Correct" <- w2
      "IT-Success" <- w2
      "IT-Total" <- w2
      "IT-%Correct" <- w2
      "MT-Success" <- w2
      "MT-Total" <- w2
      "MT-%Correct" <- w2
      "IMT-Success" <- w2
      "IMT-Total" <- w2
      "IMT-%Correct" <- w2
      "#SuccessfulBlockTrials" <- w1
    }
    frame #1 {
      n64 = stacked-sequence {
        frame #0 {
          n65 = disable-structure shown="Disabled" {
            frame Disabled {
              # "Get Host Time and Sync with RT"
              n66 = local read "GetHostTimeVI"() -> (w116:path)
              n67 = Open Application Reference(10:u16 3362 ("port number or service name (3363)"), 11:"155.101.184.21" ("machine name (\"\":  open local reference)")) -> (0:w109:errorcluster, 3:w106:refnum<vi>)  [unwired: 2 in]
              n68 = Open VI Reference(type specifier VI Refnum (for type only)=refnum<vi> refnum, application reference (local)=w106, vi path=w116, error in (no error)=w109) -> (vi reference=w108:refnum<vi>, error out=w110:errorcluster)  [unwired: 2 in]
              n69 = call-by-ref "?"(reference=w108, error in=w110) -> (error out=w112:errorcluster, "current time"=w111:timestamp)  [unwired: 1 in, 1 out]
              n70 = call <vilib>:"Initialize Session.vi"("Target (localhost)"=refnum<k21> "localhost" ("target (localhost)")) -> ("Session out"=w114:refnum<k21>)  [unwired: 9 in, 1 out]
              n71 = call <vilib>:"Set Time.vi"("error in (no error)"=w112, "Time"=w111, "Session in (localhost)"=w114) -> ("error out"=w113:errorcluster)  [unwired: 5 in, 3 out]
              n72 = call <vilib>:"Simple Error Handler.vi"("error in (no error)"=w113) -> ()  [unwired: 4 in, 5 out]
            }
            frame Enabled {
            }
          }
        }
        frame #1 {
          n73 = call "UpdateDatabaseRemote.vi"("CallType"=enum16{"Initialize", "Save", "Load"}."Initialize") -> ("ExperimentDatesSorted"=w117:string[])  [unwired: 2 in, 2 out]
          n74 = property on="RecordsSelection" class="CmbBox"("Text.Text"="") -> ()  [unwired: 2 in, 2 out]
          n75 = property on="RecordsSelection" class="CmbBox"("Strings[]"=w117) -> ()  [unwired: 2 in, 2 out]
          n76 = local write "Database"(T18 {"ExperimentDate"=timestamp(3488537986.592 s since 1904-01-01), "ImplantDate"=timestamp(-9593222400 s since 1904-01-01), "CerebusFolder"="20130416-162600", "Experimenter"="Cody Barton", "NHP Name"="Frak", "DeviceType"="USEA", "DeviceSerial"="8049-000002", "DeviceHemisphere"="Right", "DeviceRegion"="Median Nerve", "TaskType"="FingerMove.vi", "TaskComments"="", "RecordingComments"="", "GeneralObservations"=""} ("Database")) -> ()
        }
        frame #2 {
          n77 = Two Button Dialog(message="Automatically start Central recording?\nIf not, manually start recording now.", 1:"No" ("T button name (\"OK\")"), 2:"Yes" ("T button name (\"OK\")")) -> (T button?=w124:bool)
          n78 = case shown="True" w124 {
            frame False {
              n79 = local write "StopRecording"(FALSE ("StopRecording")) -> ()
            }
            frame True {
              n80 = local read "AutoCentraVI"() -> (w131:path)
              n81 = Open Application Reference(10:u16 3362 ("port number or service name (3363)"), 11:"192.168.0.1" ("machine name (\"\":  open local reference)")) -> (0:w134:errorcluster, 3:w136:refnum<vi>)  [unwired: 2 in]
              n82 = Open VI Reference(type specifier VI Refnum (for type only)=refnum<vi> refnum, application reference (local)=w136, vi path=w131, error in (no error)=w134) -> (vi reference=w132:refnum<vi>, error out=w133:errorcluster)  [unwired: 2 in]
              n83 = local read "CerebusConfigFile"() -> (w126:path)
              n84 = Get Date/Time In Seconds() -> (seconds since 1Jan1904=w130:timestamp)
              n85 = local write "StopRecording"(TRUE ("StopRecording")) -> ()
              n86 = call-by-ref "?"(reference=w132, error in=w133, "ConfigurationFile"=w126, "Mode"=T19."StartRecording") -> ("DataFolder"=w127:string, "Recording?"=w128:bool)  [unwired: 1 in, 3 out]
              n87 = local write "StartTime"(w130) -> ()
              n88 = local write "Recording?"(w128) -> ()
              n89 = local write "CerebusFolder"(w127) -> ()
            }
          }
        }
      }
      n90 = stacked-sequence {
        frame #0 {
          # "Sets motor output to 20% (1-dutycycle)"
          # "Moves actuator outward"
          n91 = local read "PWMFreq(Hz)"() -> (w140:dbl)
          n92 = local read "PWMTaskA"() -> (w147:refnum<k21>)
          n93 = local read "PWMTaskC"() -> (w141:refnum<k21>)
          n94 = local read "PWMTaskB"() -> (w144:refnum<k21>)
          n95 = call-poly <vilib>:"DAQmx Write.vi"("task/channels in"=w141, "frequency"=w140, "duty cycle"=0.8) -> ()  [unwired: 10 in, 3 out]
          n96 = call-poly <vilib>:"DAQmx Write.vi"("task/channels in"=w147, "frequency"=w140, "duty cycle"=0.8) -> ()  [unwired: 10 in, 3 out]
          n97 = call-poly <vilib>:"DAQmx Write.vi"("task/channels in"=w144, "frequency"=w140, "duty cycle"=0.8) -> ()  [unwired: 10 in, 3 out]
          n98 = call-poly <vilib>:"DAQmx Write.vi"("task/channels in"=refnum<k21> "MotorDirABC", "data"=bool[] [FALSE, FALSE, FALSE]) -> ()  [unwired: 11 in, 3 out]
        }
        frame #1 {
          n99 = Wait (ms)(milliseconds to wait=u32 2000) -> ()  [unwired: 1 out]
        }
        frame #2 {
          # "Restarts the encoder task to acquire a zero\nstarting position (actuator fully out)"
          n100 = call <vilib>:"DAQmx Stop Task.vi"("task/channels in"=refnum<k21> "PositionInA") -> ("task out"=w159:refnum<k21>, "error out"=w158:errorcluster)  [unwired: 13 in]
          n101 = call <vilib>:"DAQmx Stop Task.vi"("task/channels in"=refnum<k21> "PositionInB") -> ("task out"=w156:refnum<k21>, "error out"=w157:errorcluster)  [unwired: 13 in]
          n102 = call <vilib>:"DAQmx Stop Task.vi"("task/channels in"=refnum<k21> "PositionInC") -> ("task out"=w151:refnum<k21>, "error out"=w150:errorcluster)  [unwired: 13 in]
          n103 = call <vilib>:"DAQmx Start Task.vi"("task/channels in"=w159, "error in"=w158) -> ("error out"=w161:errorcluster)  [unwired: 12 in, 1 out]
          n104 = call <vilib>:"DAQmx Start Task.vi"("task/channels in"=w156, "error in"=w157) -> ("error out"=w154:errorcluster)  [unwired: 12 in, 1 out]
          n105 = call <vilib>:"DAQmx Start Task.vi"("task/channels in"=w151, "error in"=w150) -> ("error out"=w153:errorcluster)  [unwired: 12 in, 1 out]
          n106 = call <vilib>:"General Error Handler.vi"("error in (no error)"=w161) -> ()  [unwired: 10 in, 5 out]
          n107 = call <vilib>:"General Error Handler.vi"("error in (no error)"=w154) -> ()  [unwired: 10 in, 5 out]
          n108 = call <vilib>:"General Error Handler.vi"("error in (no error)"=w153) -> ()  [unwired: 10 in, 5 out]
        }
        frame #3 {
          # "Reverses motor direction so actuator moves\ninward"
          n109 = call-poly <vilib>:"DAQmx Write.vi"("task/channels in"=refnum<k21> "MotorDirABC", "data"=bool[] [TRUE, TRUE, TRUE]) -> ()  [unwired: 11 in, 3 out]
        }
        frame #4 {
          n110 = Wait (ms)(milliseconds to wait=u32 2000) -> ()  [unwired: 1 out]
        }
        frame #5 {
          # "Records maximum inward actuator position"
          n111 = call-poly <vilib>:"DAQmx Read.vi"("task/channels in"=refnum<k21> "PositionInA") -> ("data"=w168:dbl)  [unwired: 12 in, 2 out]
          n112 = call-poly <vilib>:"DAQmx Read.vi"("task/channels in"=refnum<k21> "PositionInB") -> ("data"=w167:dbl)  [unwired: 12 in, 2 out]
          n113 = call-poly <vilib>:"DAQmx Read.vi"("task/channels in"=refnum<k21> "PositionInC") -> ("data"=w166:dbl)  [unwired: 12 in, 2 out]
          n114 = Build Array(w168, w167, w166) -> (w165:dbl[])
          n115 = local write "EncMax"(w165) -> ()
        }
        frame #6 {
          # "Sets motor output to minimum"
          n116 = local read "PWMFreq(Hz)"() -> (w172:dbl)
          n117 = local read "PWMTaskA"() -> (w177:refnum<k21>)
          n118 = local read "PWMTaskC"() -> (w173:refnum<k21>)
          n119 = local read "PWMTaskB"() -> (w176:refnum<k21>)
          n120 = call-poly <vilib>:"DAQmx Write.vi"("task/channels in"=w177, "frequency"=w172, "duty cycle"=0.999) -> ()  [unwired: 10 in, 3 out]
          n121 = call-poly <vilib>:"DAQmx Write.vi"("task/channels in"=w173, "frequency"=w172, "duty cycle"=0.999) -> ()  [unwired: 10 in, 3 out]
          n122 = call-poly <vilib>:"DAQmx Write.vi"("task/channels in"=w176, "frequency"=w172, "duty cycle"=0.999) -> ()  [unwired: 10 in, 3 out]
        }
      }
    }
    frame #2 {
      n123 = node-c288() -> (w181:T20)  [unwired: 4 in]
      n124 = local read "PIDLoopFreq(Hz)"() -> (w179:dbl)
      n125 = timed-loop {
        timing: w181 -> [_]
        timing-out: [_] -> w180
        i -> [w232]
        stop <- w231 stop-if-true
        n126 = node-c288() -> (w227:bool, w229:i64, w225:i64)  [unwired: 1 in]
        n127 = local read "Vis_Center_Y"() -> (w190:dbl)
        n128 = local read "DrawSize"() -> (w195:T2)
        n129 = Cluster To Array(cluster=w195) -> (array=w194:u32[])
        n130 = local read "Vis_Center X"() -> (w200:dbl)
        n131 = local read "Scalefactor"() -> (w209:dbl)
        n132 = local read "DrawSize 2"() -> (w215:T2)
        n133 = local read "TargetPos"() -> (w221:dbl[])
        n134 = local read "DrawSize"() -> (w217:T2)
        n135 = local read "EncMax"() -> (w214:dbl[])
        n136 = local read "Blank 2"() -> (w216:picture)
        n137 = local read "EncPos"() -> (w224:cluster{"[0]":dbl, "[1]":dbl, "[2]":dbl})
        n138 = Index Array(array=w194) -> (element #1=w192:u32, element #2=w193:u32)  [unwired: 2 in]
        n139 = local read "Radius"() -> (w213:dbl)
        n140 = local read "MultR"() -> (w210:dbl)
        n141 = local read "Blank"() -> (w218:picture)
        n142 = Divide(x=w193, y=w192) -> (x/y=w191:dbl)
        n143 = local read "InitialPos"() -> (w204:dbl[])
        n144 = Cluster To Array(cluster=w224) -> (array=w222:dbl[])
        n145 = Multiply(x=w209, y=w210) -> (x*y=w208:dbl)
        n146 = Multiply(x=w190, y=w191) -> (x*y=w189:dbl)
        n147 = Index Array(array=w214) -> (element=w212:dbl)  [unwired: 1 in]
        n148 = Divide(x=w221, y=w214) -> (x/y=w202:dbl[])
        n149 = Replace Array Subset(array=dbl[] [0.7, 0.6, 0.7], new element #1=w200, index #1=0, new element #2=w189, index #2=2) -> (w197:dbl[])
        n150 = Divide(x=w222, y=w214) -> (x/y=w203:dbl[])
        n151 = local read "Middle Reverse Mode"() -> (w188:bool)
        n152 = Divide(x=w213, y=w212) -> (x/y=w220:dbl)
        n153 = Subtract(x=w204, y=w197) -> (x-y=w196:dbl[])
        n154 = local write "LoopCount"(w232) -> ()
        n155 = local read "RecordsSelection"() -> (w206:string)
        n156 = Subtract(x=w203, y=w196) -> (x-y=w186:dbl[])
        n157 = Subtract(x=w202, y=w196) -> (x-y=w187:dbl[])
        n158 = feedback #1(w206) -> (w207:string)
        n159 = feedback-in #1(w206) -> ()
        n160 = case shown="True" w188 {
          tunnel: w186 -> [w233 w245]
          tunnel: [w233 w242] -> w185
          frame False {
          }
          frame True {
            # "Middle Reversal mode is a training mode\nspecifically meant for Izzle.  It subtracts \nthe middle finger position from the index\nfinger position, making it impossible to \nmove the cursor towards the target when\npulling on both levers."
            n161 = local read "InitialPos"() -> (w234:dbl[])
            n162 = local read "EncMax"() -> (w239:dbl[])
            n163 = local read "EncPos"() -> (w238:cluster{"[0]":dbl, "[1]":dbl, "[2]":dbl})
            n164 = Index Array(array=w245, index=0) -> (element=w246:dbl)
            n165 = Cluster To Array(cluster=w238) -> (array=w237:dbl[])
            n166 = Divide(x=w237, y=w239) -> (x/y=w240:dbl[])
            n167 = Subtract(x=w240, y=w234) -> (x-y=w241:dbl[])
            n168 = Index Array(array=w241, index=1) -> (element=w235:dbl)
            n169 = Subtract(x=w246, y=w235) -> (x-y=w244:dbl)
            n170 = Replace Array Subset(array=w245, new element=w244, index=0) -> (w242:dbl[])
          }
        }
        n171 = Divide(x=w229, y=i64 1000) -> (x/y=w226:dbl)
        n172 = Equal?(x=w206, y=w207) -> (x = y?=w205:bool)
        n173 = case shown="False" w205 {
          frame False {
            n174 = local read "RecordsSelection"() -> (w250:string)
            n175 = call "UpdateDatabaseRemote.vi"("RecordsSelection"=w250, "CallType"=enum16{"Initialize", "Save", "Load"}."Load") -> ("DatabaseOut"=w248:T14)  [unwired: 1 in, 2 out]
            n176 = local write "Database"(w248) -> ()
          }
          frame True {
          }
        }
        n177 = local write "LoopTime"(w225) -> ()
        n178 = local write "SlowLoop"(w227) -> ()
        n179 = local write "LoopPeriod"(w226) -> ()
        n180 = call "InWindow3D.vi"("Radius"=w220, "TargXYZ"=w187, "PosXYZ"=w185) -> ("Status"=w211:enum16{"In", "Out"})  [unwired: 1 in]
        n181 = call "Disp3D.vi"("Status"=w211, "MultR"=w208, "TargXYZ"=w187, "PosXYZ"=w185, "DrawSize"=w215, "Blank"=w216) -> ("Pic"=w219:picture)
        n182 = call "Disp3D.vi"("Status"=w211, "MultR"=w210, "TargXYZ"=w187, "PosXYZ"=w185, "DrawSize"=w217, "Blank"=w218) -> ("Pic"=w223:picture)
        n183 = local read "Current State"() -> (w230:T13)
        n184 = local write "Display 2"(w219) -> ()
        n185 = local write "Display"(w223) -> ()
        n186 = local write "Status"(w211) -> ()
        n187 = case shown="\"Finalize\"" w230 {
          frame "Initialize", Default {
            n188 = local read "LoopCount"() -> (w256:u64)
            n189 = local read "InitialForce"() -> (w259:dbl[])
            n190 = local read "InitialPos"() -> (w253:dbl[])
            n191 = local read "EncMax"() -> (w252:dbl[])
            n192 = call "LoopComp.vi"("LoopCount"=w256, "Instance"=0, "Mode"=enum16{"Reset", "Run"}."Reset") -> ()  [unwired: 3 in, 2 out]
            n193 = local write "SetPoint"(w259) -> ()
            n194 = local write "Current State"(T13."Acquire Start" ("Current State")) -> ()
            n195 = local write "Finalize"(enum16{"Reward", "Cerebus", "Reset"}."Reward" ("Finalize")) -> ()
            n196 = Multiply(x=w253, y=w252) -> (x*y=w251:dbl[])
            n197 = local write "TargetPos"(w251) -> ()
            n198 = call "RunOnce.vi"("Instance"=0, "Mode"=enum16{"Reset", "Run"}."Reset") -> ()  [unwired: 1 out]
          }
          frame "Acquire Start" {
            n199 = local read "Pause"() -> (w262:bool)
            n200 = case shown="False" w262 {
              frame False {
                n201 = local read "Status"() -> (w263:enum16{"In", "Out"})
                n202 = case shown="\"In\"" w263 {
                  frame "In" {
                    n203 = local read "Timing"() -> (w265:T15)
                    n204 = local read "LoopPeriod"() -> (w271:u64)
                    n205 = local read "LoopCount"() -> (w268:u64)
                    n206 = Unbundle By Name(w265) -> ("ASD"=w264:dbl)
                    n207 = call "LoopComp.vi"("RandTime"=u64 200, "LoopPeriod"=w271, "SetTime"=w264, "LoopCount"=w268, "Instance"=0, "Mode"=enum16{"Reset", "Run"}."Run") -> ("Outcome"=w266:enum16{"TimeIn", "TimeOut"})  [unwired: 1 out]
                    n208 = case shown="\"TimeOut\"" w266 {
                      frame "TimeIn", Default {
                      }
                      frame "TimeOut" {
                        n209 = local read "RandFinger"() -> (w298:bool)
                        n210 = case shown="True" w298 {
                          frame False {
                            w303 = 0
                            n211 = local read "Displacement"() -> (w312:dbl[])
                            n212 = local read "InitialPos"() -> (w306:dbl[])
                            n213 = local read "Finger"() -> (w314:T3)
                            n214 = local read "EncMax"() -> (w305:dbl[])
                            n215 = Cluster To Array(cluster=w314) -> (array=w308:bool[])
                            n216 = Multiply(x=w306, y=w305) -> (x*y=w304:dbl[])
                            n217 = Boolean To (0,1)(Boolean=w308) -> (0, 1=w309:i16[])
                            n218 = Boolean Array To Number(Boolean array=w308) -> (number=w307:u32)
                            n219 = Negate(x=w312) -> (-x=w313:dbl[])
                            n220 = Multiply(x=w309, y=w313) -> (x*y=w310:dbl[])
                            n221 = local write "FingerNum"(w307) -> ()
                            n222 = Add(x=w310, y=w304) -> (x+y=w311:dbl[])
                            n223 = local write "#SuccessfulBlockTrials"(w303) -> ()
                            n224 = local write "#TotalBlockTrials"(w303) -> ()
                            n225 = local write "TargetPos"(w311) -> ()
                          }
                          frame True {
                            n226 = local read "#SuccessfulBlockTrials"() -> (w317:u16)
                            n227 = local read "#TotalBlockTrials"() -> (w318:u16)
                            n228 = local read "Rand_BlockSize"() -> (w320:u16)
                            n229 = Greater Or Equal?(x=w317, y=w320) -> (x >= y?=w316:bool)
                            n230 = Equal To 0?(x=w318) -> (x = 0?=w315:bool)
                            n231 = Or(x=w316, y=w315) -> (x .or. y?=w319:bool)
                            n232 = case shown="False" w319 {
                              tunnel: [w339 w341] -> w321
                              tunnel: w318 -> [w338 _]
                              frame False {
                                n233 = Increment(x=w338) -> (x+1=w337:u16)
                                n234 = local read "FingerNum"() -> (w339:dbl)
                                n235 = local write "#TotalBlockTrials"(w337) -> ()
                              }
                              frame True {
                                n236 = local read "Thumb-Success"() -> (w345:dbl)
                                n237 = local read "Middle-Success"() -> (w347:dbl)
                                n238 = local read "Index-Success"() -> (w348:dbl)
                                n239 = local read "IMT-Success"() -> (w342:dbl)
                                n240 = local read "MT-Success"() -> (w343:dbl)
                                n241 = local read "IM-Success"() -> (w346:dbl)
                                n242 = local read "IT-Success"() -> (w344:dbl)
                                n243 = local write "#SuccessfulBlockTrials"(0) -> ()
                                n244 = local write "#TotalBlockTrials"(1) -> ()
                                n245 = call "SelectFingerMovement.vi"("I_#success"=w348, "M_#success"=w347, "IM_#success"=w346, "T_#success"=w345, "IT_#success"=w344, "MT_#success"=w343, "IMT_#success"=w342) -> ("Finger_Number"=w341:dbl)  [unwired: 20 in]
                              }
                            }
                            n246 = Number To Boolean Array(number=w321) -> (Boolean array=w332:bool[])
                            n247 = local write "FingerNum"(w321) -> ()
                            n248 = Index Array(array=w332) -> (element #1=w335:bool, element #2=w333:bool, element #3=w334:bool)  [unwired: 3 in]
                            n249 = local read "Finger"() -> (w336:T3)
                            n250 = local read "Displacement"() -> (w330:dbl[])
                            n251 = Bundle By Name(cluster=w336, "Index"=w335, "Middle"=w333, "Thumb"=w334) -> (w325:T3)
                            n252 = local read "InitialPos"() -> (w324:dbl[])
                            n253 = local read "EncMax"() -> (w323:dbl[])
                            n254 = Cluster To Array(cluster=w325) -> (array=w326:bool[])
                            n255 = Boolean To (0,1)(Boolean=w326) -> (0, 1=w327:i16[])
                            n256 = Negate(x=w330) -> (-x=w331:dbl[])
                            n257 = Multiply(x=w324, y=w323) -> (x*y=w322:dbl[])
                            n258 = Multiply(x=w327, y=w331) -> (x*y=w328:dbl[])
                            n259 = Add(x=w328, y=w322) -> (x+y=w329:dbl[])
                            n260 = local write "TargetPos"(w329) -> ()
                          }
                        }
                        n261 = call "RunOnce.vi"("Instance"=0, "Mode"=enum16{"Reset", "Run"}."Reset") -> ()  [unwired: 1 out]
                        n262 = call "RunOnce.vi"("Instance"=1, "Mode"=enum16{"Reset", "Run"}."Reset") -> ()  [unwired: 1 out]
                        n263 = Open Application Reference(10:u16 3362 ("port number or service name (3363)"), 11:"192.168.0.1" ("machine name (\"\":  open local reference)")) -> (0:w294:errorcluster, 3:w295:refnum<vi>)  [unwired: 2 in]
                        n264 = Open VI Reference(type specifier VI Refnum (for type only)=refnum<vi> refnum, application reference (local)=w295, vi path=path "E:/Code/Tasks/SubVIs/playsound.vi", error in (no error)=w294) -> (vi reference=w292:refnum<vi>, error out=w291:errorcluster)  [unwired: 2 in]
                        n265 = call-by-ref "?"(reference=w292, error in=w291, "Volume"=1.0, "Mode"=enum16{"Cue", "Success", "Failure", "Abort"}."Cue", "#S"=100.0, "Fs"=5000.0) -> ()  [unwired: 8 in, 2 out]
                        n266 = local read "FingerNum"() -> (w277:dbl)
                        n267 = local read "LoopCount"() -> (w299:u64)
                        n268 = Format Into String(format string="%0.0f", w277) -> (resulting string=w274:string)  [unwired: 2 in, 1 out]
                        n269 = local read "LoopCount"() -> (w281:u64)
                        n270 = local write "Current State"(T13."Acquire Response" ("Current State")) -> ()
                        n271 = Concatenate Strings("TargOn=" ("String"), w274, ";" ("string")) -> (w276:string)
                        n272 = call "LoopComp.vi"("LoopCount"=w299, "Instance"=0, "Mode"=enum16{"Reset", "Run"}."Reset") -> ()  [unwired: 3 in, 2 out]
                        n273 = call "SendCerebus8.vi"("String"=w276, "Mode"=T16."String") -> ()  [unwired: 3 in]
                        n274 = call "LoopComp.vi"("LoopCount"=w281, "Instance"=1, "Mode"=enum16{"Reset", "Run"}."Reset") -> ()  [unwired: 3 in, 2 out]
                      }
                    }
                  }
                  frame "Out", Default {
                    n275 = local read "LoopCount"() -> (w350:u64)
                    n276 = call "LoopComp.vi"("LoopCount"=w350, "Instance"=0, "Mode"=enum16{"Reset", "Run"}."Reset") -> ()  [unwired: 3 in, 2 out]
                  }
                }
              }
              frame True {
                n277 = local read "LoopCount"() -> (w353:u64)
                n278 = call "LoopComp.vi"("LoopCount"=w353, "Instance"=0, "Mode"=enum16{"Reset", "Run"}."Reset") -> ()  [unwired: 3 in, 2 out]
              }
            }
          }
          frame "Acquire Response" {
            n279 = local read "Timing"() -> (w358:T15)
            n280 = local read "LoopPeriod"() -> (w363:u64)
            n281 = local read "LoopCount"() -> (w360:u64)
            n282 = Unbundle By Name(w358) -> ("ARD"=w357:dbl)
            n283 = call "LoopComp.vi"("RandTime"=u64 200, "LoopPeriod"=w363, "SetTime"=w357, "LoopCount"=w360, "Instance"=0, "Mode"=enum16{"Reset", "Run"}."Run") -> ("Outcome"=w356:enum16{"TimeIn", "TimeOut"})  [unwired: 1 out]
            n284 = case shown="\"TimeIn\", Default" w356 {
              frame "TimeIn", Default {
                n285 = local read "Status"() -> (w364:enum16{"In", "Out"})
                n286 = case shown="\"Out\", Default" w364 {
                  frame "In" {
                    n287 = local read "Timing"() -> (w371:T15)
                    n288 = local read "LoopPeriod"() -> (w366:u64)
                    n289 = local read "LoopCount"() -> (w369:u64)
                    n290 = Unbundle By Name(w371) -> ("HoldTime"=w372:dbl)
                    n291 = call "LoopComp.vi"("RandTime"=u64 200, "LoopPeriod"=w366, "SetTime"=w372, "LoopCount"=w369, "Instance"=1, "Mode"=enum16{"Reset", "Run"}."Run") -> ("Outcome"=w365:enum16{"TimeIn", "TimeOut"})  [unwired: 1 out]
                    n292 = case shown="\"TimeOut\"" w365 {
                      frame "TimeIn", Default {
                        n293 = call "RunOnce.vi"("Instance"=0, "Mode"=enum16{"Reset", "Run"}."Run") -> ("State"=w375:enum16{"RunOnce", "Finished"})
                        n294 = case shown="\"RunOnce\", Default" w375 {
                          frame "RunOnce", Default {
                            n295 = local read "FingerNum"() -> (w381:dbl)
                            n296 = Format Into String(format string="%0.0f", w381) -> (resulting string=w379:string)  [unwired: 2 in, 1 out]
                            n297 = Concatenate Strings("TargIn=" ("String"), w379, ";" ("string")) -> (w380:string)
                            n298 = call "SendCerebus8.vi"("String"=w380, "Mode"=T16."String") -> ()  [unwired: 3 in]
                          }
                          frame "Finished" {
                          }
                        }
                      }
                      frame "TimeOut" {
                        n299 = local read "FingerNum"() -> (w391:dbl)
                        n300 = local read "InitialPos"() -> (w385:dbl[])
                        n301 = local read "EncMax"() -> (w384:dbl[])
                        n302 = Format Into String(format string="%0.0f", w391) -> (resulting string=w388:string)  [unwired: 2 in, 1 out]
                        n303 = Multiply(x=w385, y=w384) -> (x*y=w383:dbl[])
                        n304 = Concatenate Strings("TargAcq=" ("String"), w388, ";" ("string")) -> (w390:string)
                        n305 = local read "LoopCount"() -> (w394:u64)
                        n306 = local write "TargetPos"(w383) -> ()
                        n307 = call "SendCerebus8.vi"("String"=w390, "Mode"=T16."String") -> ()  [unwired: 3 in]
                        n308 = local write "Outcome"("Success" ("Outcome")) -> ()
                        n309 = local write "Current State"(T13."Finalize" ("Current State")) -> ()
                        n310 = call "LoopComp.vi"("LoopCount"=w394, "Instance"=0, "Mode"=enum16{"Reset", "Run"}."Reset") -> ()  [unwired: 3 in, 2 out]
                        n311 = call "RunOnce.vi"("Instance"=0, "Mode"=enum16{"Reset", "Run"}."Reset") -> ()  [unwired: 1 out]
                      }
                    }
                  }
                  frame "Out", Default {
                    n312 = local read "InitialPos"() -> (w402:dbl[])
                    n313 = local read "EncMax"() -> (w401:dbl[])
                    n314 = Multiply(x=w402, y=w401) -> (x*y=w400:dbl[])
                    n315 = local read "TrainThresh"() -> (w403:dbl[])
                    n316 = local read "EncPos"() -> (w413:cluster{"[0]":dbl, "[1]":dbl, "[2]":dbl})
                    n317 = local read "TargetPos"() -> (w415:dbl[])
                    n318 = Subtract(x=w400, y=w415) -> (x-y=w414:dbl[])
                    n319 = Cluster To Array(cluster=w413) -> (array=w409:dbl[])
                    n320 = Add(x=w414, y=w403) -> (x+y=w404:dbl[])
                    n321 = Add(x=w400, y=w404) -> (x+y=w410:dbl[])
                    n322 = Subtract(x=w400, y=w404) -> (x-y=w412:dbl[])
                    n323 = Greater?(x=w409, y=w412) -> (0:w411:bool[])
                    n324 = Less?(x=w409, y=w410) -> (x < y?=w408:bool[])
                    n325 = And Array Elements(Boolean array=w408) -> (logical AND=w407:bool)
                    n326 = And Array Elements(Boolean array=w411) -> (logical AND=w406:bool)
                    n327 = And(x=w407, y=w406) -> (x .and. y?=w405:bool)
                    n328 = case shown="False" w405 {
                      frame False {
                        n329 = local read "LoopCount"() -> (w420:u64)
                        n330 = local write "Outcome"("Failure" ("Outcome")) -> ()
                        n331 = local write "Current State"(T13."Finalize" ("Current State")) -> ()
                        n332 = call "LoopComp.vi"("LoopCount"=w420, "Instance"=0, "Mode"=enum16{"Reset", "Run"}."Reset") -> ()  [unwired: 3 in, 2 out]
                        n333 = call "RunOnce.vi"("Instance"=0, "Mode"=enum16{"Reset", "Run"}."Reset") -> ()  [unwired: 1 out]
                      }
                      frame True {
                        n334 = local read "LoopCount"() -> (w423:u64)
                        n335 = call "LoopComp.vi"("LoopCount"=w423, "Instance"=1, "Mode"=enum16{"Reset", "Run"}."Reset") -> ()  [unwired: 3 in, 2 out]
                      }
                    }
                  }
                }
              }
              frame "TimeOut" {
                n336 = local read "LoopCount"() -> (w430:u64)
                n337 = local write "Outcome"("Abort" ("Outcome")) -> ()
                n338 = local write "Current State"(T13."Finalize" ("Current State")) -> ()
                n339 = call "RunOnce.vi"("Instance"=0, "Mode"=enum16{"Reset", "Run"}."Reset") -> ()  [unwired: 1 out]
                n340 = call "LoopComp.vi"("LoopCount"=w430, "Instance"=0, "Mode"=enum16{"Reset", "Run"}."Reset") -> ()  [unwired: 3 in, 2 out]
              }
            }
          }
          frame "Finalize" {
            n341 = local read "Finalize"() -> (w433:enum16{"Reward", "Cerebus", "Reset"})
            n342 = case shown="\"Cerebus\"" w433 {
              frame "Reward", Default {
                n343 = local read "Outcome"() -> (w434:string)
                n344 = case shown="\"Success\"" w434 {
                  frame "Abort", Default {
                    n345 = local read "Timing"() -> (w436:T15)
                    n346 = local read "LoopPeriod"() -> (w442:u64)
                    n347 = local read "LoopCount"() -> (w439:u64)
                    n348 = Unbundle By Name(w436) -> ("AbortTime"=w435:dbl)
                    n349 = call "LoopComp.vi"("RandTime"=u64 200, "LoopPeriod"=w442, "SetTime"=w435, "LoopCount"=w439, "Instance"=0, "Mode"=enum16{"Reset", "Run"}."Run") -> ("Outcome"=w438:enum16{"TimeIn", "TimeOut"})  [unwired: 1 out]
                    n350 = case shown="\"TimeOut\"" w438 {
                      frame "TimeIn", Default {
                        n351 = Build Array(10, 10, 10) -> (w443:i32[])
                        n352 = local write "TargetPos"(w443) -> ()
                        n353 = call "RunOnce.vi"("Instance"=0, "Mode"=enum16{"Reset", "Run"}."Run") -> ("State"=w447:enum16{"RunOnce", "Finished"})
                        n354 = case shown="\"RunOnce\", Default" w447 {
                          frame "RunOnce", Default {
                            n355 = Open Application Reference(10:u16 3362 ("port number or service name (3363)"), 11:"192.168.0.1" ("machine name (\"\":  open local reference)")) -> (0:w458:errorcluster, 3:w459:refnum<vi>)  [unwired: 2 in]
                            n356 = Open VI Reference(type specifier VI Refnum (for type only)=refnum<vi> refnum, application reference (local)=w459, vi path=path "E:/Code/PID/SubVIs/playsound.vi", error in (no error)=w458) -> (vi reference=w456:refnum<vi>, error out=w455:errorcluster)  [unwired: 2 in]
                            n357 = call-by-ref "?"(reference=w456, error in=w455, "Volume"=1.0, "Mode"=enum16{"Cue", "Success", "Failure", "Abort"}."Abort", "#S"=1000.0, "Fs"=5000.0) -> ()  [unwired: 8 in, 2 out]
                          }
                          frame "Finished" {
                          }
                        }
                      }
                      frame "TimeOut" {
                        n358 = local read "FingerNum"() -> (w462:dbl)
                        n359 = local read "InitialPos"() -> (w470:dbl[])
                        n360 = local read "EncMax"() -> (w469:dbl[])
                        n361 = case shown="7" w462 {
                          frame 3 {
                            n362 = local read "IM-Success"() -> (w476:dbl)
                            n363 = local read "IM-Total"() -> (w481:dbl)
                            n364 = Increment(x=w481) -> (x+1=w480:dbl)
                            n365 = Divide(x=w476, y=w480) -> (x/y=w479:dbl)
                            n366 = Multiply(x=w479, y=100.0) -> (x*y=w477:dbl)
                            n367 = local write "IM-Total"(w480) -> ()
                            n368 = local write "IM-%Correct"(w477) -> ()
                          }
                          frame 4 {
                            n369 = local read "Thumb-Success"() -> (w482:dbl)
                            n370 = local read "Thumb-Total"() -> (w487:dbl)
                            n371 = Increment(x=w487) -> (x+1=w486:dbl)
                            n372 = Divide(x=w482, y=w486) -> (x/y=w485:dbl)
                            n373 = Multiply(x=w485, y=100.0) -> (x*y=w483:dbl)
                            n374 = local write "Thumb-Total"(w486) -> ()
                            n375 = local write "Thumb-%Correct"(w483) -> ()
                          }
                          frame 5 {
                            n376 = local read "IT-Success"() -> (w488:dbl)
                            n377 = local read "IT-Total"() -> (w493:dbl)
                            n378 = Increment(x=w493) -> (x+1=w492:dbl)
                            n379 = Divide(x=w488, y=w492) -> (x/y=w491:dbl)
                            n380 = Multiply(x=w491, y=100.0) -> (x*y=w489:dbl)
                            n381 = local write "IT-Total"(w492) -> ()
                            n382 = local write "IT-%Correct"(w489) -> ()
                          }
                          frame 6 {
                            n383 = local read "MT-Success"() -> (w494:dbl)
                            n384 = local read "MT-Total"() -> (w499:dbl)
                            n385 = Increment(x=w499) -> (x+1=w498:dbl)
                            n386 = Divide(x=w494, y=w498) -> (x/y=w497:dbl)
                            n387 = Multiply(x=w497, y=100.0) -> (x*y=w495:dbl)
                            n388 = local write "MT-Total"(w498) -> ()
                            n389 = local write "MT-%Correct"(w495) -> ()
                          }
                          frame 7 {
                            n390 = local read "IMT-Success"() -> (w500:dbl)
                            n391 = local read "IMT-Total"() -> (w505:dbl)
                            n392 = Increment(x=w505) -> (x+1=w504:dbl)
                            n393 = Divide(x=w500, y=w504) -> (x/y=w503:dbl)
                            n394 = Multiply(x=w503, y=100.0) -> (x*y=w501:dbl)
                            n395 = local write "IMT-Total"(w504) -> ()
                            n396 = local write "IMT-%Correct"(w501) -> ()
                          }
                          frame 1, Default {
                            n397 = local read "Index-Success"() -> (w506:dbl)
                            n398 = local read "Index-Total"() -> (w511:dbl)
                            n399 = Increment(x=w511) -> (x+1=w510:dbl)
                            n400 = Divide(x=w506, y=w510) -> (x/y=w509:dbl)
                            n401 = Multiply(x=w509, y=100.0) -> (x*y=w507:dbl)
                            n402 = local write "Index-Total"(w510) -> ()
                            n403 = local write "Index-%Correct"(w507) -> ()
                          }
                          frame 2 {
                            n404 = local read "Middle-Success"() -> (w512:dbl)
                            n405 = local read "Middle - Total"() -> (w517:dbl)
                            n406 = Increment(x=w517) -> (x+1=w516:dbl)
                            n407 = Divide(x=w512, y=w516) -> (x/y=w515:dbl)
                            n408 = Multiply(x=w515, y=100.0) -> (x*y=w513:dbl)
                            n409 = local write "Middle - Total"(w516) -> ()
                            n410 = local write "Middle - %Correct"(w513) -> ()
                          }
                        }
                        n411 = local read "SuccessfulTrials"() -> (w467:dbl)
                        n412 = local read "TrialCount"() -> (w466:i32)
                        n413 = local read "AbortTrials"() -> (w472:dbl)
                        n414 = Multiply(x=w470, y=w469) -> (x*y=w468:dbl[])
                        n415 = Divide(x=w467, y=w466) -> (x/y=w465:dbl)
                        n416 = Increment(x=w472) -> (x+1=w471:dbl)
                        n417 = Multiply(x=w465, y=100.0) -> (x*y=w464:dbl)
                        n418 = local write "TargetPos"(w468) -> ()
                        n419 = local write "Finalize"(enum16{"Reward", "Cerebus", "Reset"}."Cerebus" ("Finalize")) -> ()
                        n420 = call "RunOnce.vi"("Instance"=0, "Mode"=enum16{"Reset", "Run"}."Reset") -> ()  [unwired: 1 out]
                        n421 = local write "PercentCorrect"(w464) -> ()
                        n422 = local write "AbortTrials"(w471) -> ()
                      }
                    }
                  }
                  frame "Failure" {
                    n423 = local read "Timing"() -> (w519:T15)
                    n424 = local read "LoopPeriod"() -> (w525:u64)
                    n425 = local read "LoopCount"() -> (w522:u64)
                    n426 = Unbundle By Name(w519) -> ("AbortTime"=w518:dbl)
                    n427 = call "LoopComp.vi"("RandTime"=u64 200, "LoopPeriod"=w525, "SetTime"=w518, "LoopCount"=w522, "Instance"=0, "Mode"=enum16{"Reset", "Run"}."Run") -> ("Outcome"=w521:enum16{"TimeIn", "TimeOut"})  [unwired: 1 out]
                    n428 = case shown="\"TimeOut\"" w521 {
                      frame "TimeIn", Default {
                        n429 = Build Array(10, 10, 10) -> (w526:i32[])
                        n430 = local write "TargetPos"(w526) -> ()
                        n431 = call "RunOnce.vi"("Instance"=0, "Mode"=enum16{"Reset", "Run"}."Run") -> ("State"=w530:enum16{"RunOnce", "Finished"})
                        n432 = case shown="\"Finished\"" w530 {
                          frame "RunOnce", Default {
                            n433 = Open Application Reference(10:u16 3362 ("port number or service name (3363)"), 11:"192.168.0.1" ("machine name (\"\":  open local reference)")) -> (0:w541:errorcluster, 3:w542:refnum<vi>)  [unwired: 2 in]
                            n434 = Open VI Reference(type specifier VI Refnum (for type only)=refnum<vi> refnum, application reference (local)=w542, vi path=path "E:/Code/Tasks/SubVIs/playsound.vi", error in (no error)=w541) -> (vi reference=w539:refnum<vi>, error out=w538:errorcluster)  [unwired: 2 in]
                            n435 = call-by-ref "?"(reference=w539, error in=w538, "Volume"=1.0, "Mode"=enum16{"Cue", "Success", "Failure", "Abort"}."Abort", "#S"=1000.0, "Fs"=5000.0) -> ()  [unwired: 8 in, 2 out]
                          }
                          frame "Finished" {
                          }
                        }
                      }
                      frame "TimeOut" {
                        n436 = local read "FingerNum"() -> (w545:dbl)
                        n437 = case shown="7" w545 {
                          frame 1, Default {
                            n438 = local read "Index-Success"() -> (w559:dbl)
                            n439 = local read "Index-Total"() -> (w564:dbl)
                            n440 = Increment(x=w564) -> (x+1=w563:dbl)
                            n441 = Divide(x=w559, y=w563) -> (x/y=w562:dbl)
                            n442 = Multiply(x=w562, y=100.0) -> (x*y=w560:dbl)
                            n443 = local write "Index-Total"(w563) -> ()
                            n444 = local write "Index-%Correct"(w560) -> ()
                          }
                          frame 2 {
                            n445 = local read "Middle-Success"() -> (w565:dbl)
                            n446 = local read "Middle - Total"() -> (w570:dbl)
                            n447 = Increment(x=w570) -> (x+1=w569:dbl)
                            n448 = Divide(x=w565, y=w569) -> (x/y=w568:dbl)
                            n449 = Multiply(x=w568, y=100.0) -> (x*y=w566:dbl)
                            n450 = local write "Middle - Total"(w569) -> ()
                            n451 = local write "Middle - %Correct"(w566) -> ()
                          }
                          frame 3 {
                            n452 = local read "IM-Success"() -> (w571:dbl)
                            n453 = local read "IM-Total"() -> (w576:dbl)
                            n454 = Increment(x=w576) -> (x+1=w575:dbl)
                            n455 = Divide(x=w571, y=w575) -> (x/y=w574:dbl)
                            n456 = Multiply(x=w574, y=100.0) -> (x*y=w572:dbl)
                            n457 = local write "IM-Total"(w575) -> ()
                            n458 = local write "IM-%Correct"(w572) -> ()
                          }
                          frame 4 {
                            n459 = local read "Thumb-Success"() -> (w577:dbl)
                            n460 = local read "Thumb-Total"() -> (w582:dbl)
                            n461 = Increment(x=w582) -> (x+1=w581:dbl)
                            n462 = Divide(x=w577, y=w581) -> (x/y=w580:dbl)
                            n463 = Multiply(x=w580, y=100.0) -> (x*y=w578:dbl)
                            n464 = local write "Thumb-Total"(w581) -> ()
                            n465 = local write "Thumb-%Correct"(w578) -> ()
                          }
                          frame 5 {
                            n466 = local read "IT-Success"() -> (w583:dbl)
                            n467 = local read "IT-Total"() -> (w588:dbl)
                            n468 = Increment(x=w588) -> (x+1=w587:dbl)
                            n469 = Divide(x=w583, y=w587) -> (x/y=w586:dbl)
                            n470 = Multiply(x=w586, y=100.0) -> (x*y=w584:dbl)
                            n471 = local write "IT-Total"(w587) -> ()
                            n472 = local write "IT-%Correct"(w584) -> ()
                          }
                          frame 6 {
                            n473 = local read "MT-Success"() -> (w589:dbl)
                            n474 = local read "MT-Total"() -> (w594:dbl)
                            n475 = Increment(x=w594) -> (x+1=w593:dbl)
                            n476 = Divide(x=w589, y=w593) -> (x/y=w592:dbl)
                            n477 = Multiply(x=w592, y=100.0) -> (x*y=w590:dbl)
                            n478 = local write "MT-Total"(w593) -> ()
                            n479 = local write "MT-%Correct"(w590) -> ()
                          }
                          frame 7 {
                            n480 = local read "IMT-Success"() -> (w595:dbl)
                            n481 = local read "IMT-Total"() -> (w600:dbl)
                            n482 = Increment(x=w600) -> (x+1=w599:dbl)
                            n483 = Divide(x=w595, y=w599) -> (x/y=w598:dbl)
                            n484 = Multiply(x=w598, y=100.0) -> (x*y=w596:dbl)
                            n485 = local write "IMT-Total"(w599) -> ()
                            n486 = local write "IMT-%Correct"(w596) -> ()
                          }
                        }
                        n487 = local read "InitialPos"() -> (w553:dbl[])
                        n488 = local read "EncMax"() -> (w552:dbl[])
                        n489 = local read "SuccessfulTrials"() -> (w550:dbl)
                        n490 = local read "FailureTrials"() -> (w555:dbl)
                        n491 = local read "TrialCount"() -> (w549:i32)
                        n492 = Multiply(x=w552, y=w553) -> (x*y=w551:dbl[])
                        n493 = Divide(x=w550, y=w549) -> (x/y=w548:dbl)
                        n494 = Increment(x=w555) -> (x+1=w554:dbl)
                        n495 = local write "TargetPos"(w551) -> ()
                        n496 = Multiply(x=w548, y=100.0) -> (x*y=w547:dbl)
                        n497 = call "RunOnce.vi"("Instance"=0, "Mode"=enum16{"Reset", "Run"}."Reset") -> ()  [unwired: 1 out]
                        n498 = local write "Finalize"(enum16{"Reward", "Cerebus", "Reset"}."Cerebus" ("Finalize")) -> ()
                        n499 = local write "FailureTrials"(w554) -> ()
                        n500 = local write "PercentCorrect"(w547) -> ()
                      }
                    }
                  }
                  frame "Success" {
                    n501 = local read "Timing"() -> (w602:T15)
                    n502 = local read "LoopPeriod"() -> (w608:u64)
                    n503 = local read "LoopCount"() -> (w604:u64)
                    n504 = Unbundle By Name(w602) -> ("JuiceTime"=w601:dbl)
                    n505 = call "LoopComp.vi"("RandTime"=u64 200, "LoopPeriod"=w608, "SetTime"=w601, "LoopCount"=w604, "Instance"=0, "Mode"=enum16{"Reset", "Run"}."Run") -> ("Outcome"=w607:enum16{"TimeIn", "TimeOut"})  [unwired: 1 out]
                    n506 = case shown="\"TimeOut\"" w607 {
                      frame "TimeIn", Default {
                        n507 = call-poly <vilib>:"DAQmx Write.vi"("task/channels in"=refnum<k21> "JuiceAndScreen", "data"=5.0) -> ()  [unwired: 11 in, 3 out]
                      }
                      frame "TimeOut" {
                        n508 = local read "FingerNum"() -> (w612:dbl)
                        n509 = local read "RandFinger"() -> (w611:bool)
                        n510 = local read "SuccessfulTrials"() -> (w619:dbl)
                        n511 = local read "SuccessfulTrials"() -> (w617:dbl)
                        n512 = local read "TrialCount"() -> (w616:i32)
                        n513 = case shown="7" w612 {
                          frame 1, Default {
                            n514 = local read "Index-Success"() -> (w631:dbl)
                            n515 = local read "Index-Total"() -> (w630:dbl)
                            n516 = Increment(x=w631) -> (x+1=w629:dbl)
                            n517 = Increment(x=w630) -> (x+1=w628:dbl)
                            n518 = Divide(x=w629, y=w628) -> (x/y=w627:dbl)
                            n519 = Multiply(x=w627, y=100.0) -> (x*y=w625:dbl)
                            n520 = local write "Index-Success"(w629) -> ()
                            n521 = local write "Index-Total"(w628) -> ()
                            n522 = local write "Index-%Correct"(w625) -> ()
                          }
                          frame 2 {
                            n523 = local read "Middle-Success"() -> (w638:dbl)
                            n524 = local read "Middle - Total"() -> (w637:dbl)
                            n525 = Increment(x=w638) -> (x+1=w636:dbl)
                            n526 = Increment(x=w637) -> (x+1=w635:dbl)
                            n527 = Divide(x=w636, y=w635) -> (x/y=w634:dbl)
                            n528 = Multiply(x=w634, y=100.0) -> (x*y=w632:dbl)
                            n529 = local write "Middle-Success"(w636) -> ()
                            n530 = local write "Middle - Total"(w635) -> ()
                            n531 = local write "Middle - %Correct"(w632) -> ()
                          }
                          frame 3 {
                            n532 = local read "IM-Success"() -> (w645:dbl)
                            n533 = local read "IM-Total"() -> (w644:dbl)
                            n534 = Increment(x=w645) -> (x+1=w643:dbl)
                            n535 = Increment(x=w644) -> (x+1=w642:dbl)
                            n536 = Divide(x=w643, y=w642) -> (x/y=w641:dbl)
                            n537 = Multiply(x=w641, y=100.0) -> (x*y=w639:dbl)
                            n538 = local write "IM-Success"(w643) -> ()
                            n539 = local write "IM-Total"(w642) -> ()
                            n540 = local write "IM-%Correct"(w639) -> ()
                          }
                          frame 4 {
                            n541 = local read "Thumb-Success"() -> (w652:dbl)
                            n542 = local read "Thumb-Total"() -> (w651:dbl)
                            n543 = Increment(x=w652) -> (x+1=w650:dbl)
                            n544 = Increment(x=w651) -> (x+1=w649:dbl)
                            n545 = Divide(x=w650, y=w649) -> (x/y=w648:dbl)
                            n546 = Multiply(x=w648, y=100.0) -> (x*y=w646:dbl)
                            n547 = local write "Thumb-Success"(w650) -> ()
                            n548 = local write "Thumb-Total"(w649) -> ()
                            n549 = local write "Thumb-%Correct"(w646) -> ()
                          }
                          frame 5 {
                            n550 = local read "IT-Success"() -> (w659:dbl)
                            n551 = local read "IT-Total"() -> (w658:dbl)
                            n552 = Increment(x=w659) -> (x+1=w657:dbl)
                            n553 = Increment(x=w658) -> (x+1=w656:dbl)
                            n554 = Divide(x=w657, y=w656) -> (x/y=w655:dbl)
                            n555 = Multiply(x=w655, y=100.0) -> (x*y=w653:dbl)
                            n556 = local write "IT-Success"(w657) -> ()
                            n557 = local write "IT-Total"(w656) -> ()
                            n558 = local write "IT-%Correct"(w653) -> ()
                          }
                          frame 6 {
                            n559 = local read "MT-Success"() -> (w666:dbl)
                            n560 = local read "MT-Total"() -> (w665:dbl)
                            n561 = Increment(x=w666) -> (x+1=w664:dbl)
                            n562 = Increment(x=w665) -> (x+1=w663:dbl)
                            n563 = Divide(x=w664, y=w663) -> (x/y=w662:dbl)
                            n564 = Multiply(x=w662, y=100.0) -> (x*y=w660:dbl)
                            n565 = local write "MT-Success"(w664) -> ()
                            n566 = local write "MT-Total"(w663) -> ()
                            n567 = local write "MT-%Correct"(w660) -> ()
                          }
                          frame 7 {
                            n568 = local read "IMT-Success"() -> (w673:dbl)
                            n569 = local read "IMT-Total"() -> (w672:dbl)
                            n570 = Increment(x=w673) -> (x+1=w671:dbl)
                            n571 = Increment(x=w672) -> (x+1=w670:dbl)
                            n572 = Divide(x=w671, y=w670) -> (x/y=w669:dbl)
                            n573 = Multiply(x=w669, y=100.0) -> (x*y=w667:dbl)
                            n574 = local write "IMT-Success"(w671) -> ()
                            n575 = local write "IMT-Total"(w670) -> ()
                            n576 = local write "IMT-%Correct"(w667) -> ()
                          }
                        }
                        n577 = case shown="True" w611 {
                          frame False {
                          }
                          frame True {
                            n578 = local read "#SuccessfulBlockTrials"() -> (w623:u16)
                            n579 = Increment(x=w623) -> (x+1=w624:u16)
                            n580 = local write "#SuccessfulBlockTrials"(w624) -> ()
                          }
                        }
                        n581 = Increment(x=w619) -> (x+1=w618:dbl)
                        n582 = Divide(x=w617, y=w616) -> (x/y=w615:dbl)
                        n583 = local write "SuccessfulTrials"(w618) -> ()
                        n584 = Multiply(x=w615, y=100.0) -> (x*y=w614:dbl)
                        n585 = local write "PercentCorrect"(w614) -> ()
                        n586 = call-poly <vilib>:"DAQmx Write.vi"("task/channels in"=refnum<k21> "JuiceAndScreen", "data"=0.0) -> ()  [unwired: 11 in, 3 out]
                        n587 = local write "Finalize"(enum16{"Reward", "Cerebus", "Reset"}."Cerebus" ("Finalize")) -> ()
                      }
                    }
                  }
                }
              }
              frame "Cerebus" {
                w677 = enum16{"Normal", "Matlab"}."Matlab" ("Type")
                w678 = "%0.0f" ("Key Word")
                # "FingerNum\nInitial Position\nDisplacement\nRadius\nTrainThresh\nTiming(ASD, ARD, Hold Time)\nInitial Force\nOutcome"
                # "*TrialParameters: TrialType=Index;FingerThreshold=0.5; ...#\n*1=On#\n*1=CrossedThreshold#\n*1=Acquired#\n\nNOTE: 1 is the # from index,middle,thumb boolean array"
                n588 = local read "InitialPos"() -> (w676:dbl[])
                n589 = local read "Timing"() -> (w696:T15)
                n590 = local read "EncMax"() -> (w675:dbl[])
                n591 = Unbundle By Name(w696) -> ("ARD"=w688:dbl, "HoldTime"=w687:dbl)
                n592 = Multiply(x=w676, y=w675) -> (x*y=w674:dbl[])
                n593 = local read "Displacement"() -> (w684:dbl[])
                n594 = local read "TrainThresh"() -> (w683:dbl[])
                n595 = local read "FingerNum"() -> (w707:dbl)
                n596 = local read "InitialForce"() -> (w680:dbl[])
                n597 = local read "TrialCount"() -> (w702:i32)
                n598 = local read "Outcome"() -> (w697:string)
                n599 = local read "Radius"() -> (w686:dbl)
                n600 = call-poly "VariablesToString.vi"("ValueIn"=w697, "FieldName"="Outcome", "Type"=w677) -> ("StringOut"=w692:string)  [unwired: 4 in]
                n601 = call-poly "VariablesToString.vi"("Format"=w678, "ValueIn"=w702, "FieldName"="TrialCount" ("Key Word"), "Type"=w677) -> ("StringOut"=w691:string)  [unwired: 3 in]
                n602 = call-poly "VariablesToString.vi"("Format"=w678, "ValueIn"=w707, "FieldName"="TrialType" ("Key Word"), "Type"=w677) -> ("StringOut"=w706:string)  [unwired: 3 in]
                n603 = call-poly "VariablesToString.vi"("ValueIn"=w674, "FieldName"="InitialPosition" ("Key Word"), "Type"=w677) -> ("StringOut"=w704:string)  [unwired: 4 in]
                n604 = call-poly "VariablesToString.vi"("ValueIn"=w683, "FieldName"="TrainThresh" ("Key Word"), "Type"=w677) -> ("StringOut"=w699:string)  [unwired: 4 in]
                n605 = call-poly "VariablesToString.vi"("ValueIn"=w684, "FieldName"="Displacement" ("Key Word"), "Type"=w677) -> ("StringOut"=w698:string)  [unwired: 4 in]
                n606 = call-poly "VariablesToString.vi"("ValueIn"=w686, "FieldName"="Radius" ("Key Word"), "Type"=w677) -> ("StringOut"=w695:string)  [unwired: 4 in]
                n607 = call-poly "VariablesToString.vi"("ValueIn"=w688, "FieldName"="ARD" ("Key Word"), "Type"=w677) -> ("StringOut"=w694:string)  [unwired: 4 in]
                n608 = call-poly "VariablesToString.vi"("ValueIn"=w687, "FieldName"="HoldTime" ("Key Word"), "Type"=w677) -> ("StringOut"=w693:string)  [unwired: 4 in]
                n609 = call-poly "VariablesToString.vi"("ValueIn"=w680, "FieldName"="InitalForce", "Type"=w677) -> ("StringOut"=w700:string)  [unwired: 4 in]
                n610 = Concatenate Strings("TrialParameters:" ("string"), w706, w704, w700, w699, w698, w695, w694, w693, w692, w691) -> (w710:string)
                n611 = call "SendCerebus8.vi"("String"=w710, "Mode"=T16."String") -> ()  [unwired: 3 in]
                n612 = local write "Finalize"(enum16{"Reward", "Cerebus", "Reset"}."Reset" ("Finalize")) -> ()
              }
              frame "Reset" {
                n613 = local read "TrialCount"() -> (w715:i32)
                n614 = Increment(x=w715) -> (x+1=w714:i32)
                n615 = local write "Outcome"("--" ("Outcome")) -> ()
                n616 = local write "Current State"(T13."Initialize" ("Current State")) -> ()
                n617 = local write "TrialCount"(w714) -> ()
              }
            }
          }
        }
        n618 = local read "Stop"() -> (w231:bool)
        n619 = node-c288() -> ()  [unwired: 1 in, 1 out]
      }
      n620 = expression code="(1/x)*1e6"(w179) -> (w182:dbl)
      n621 = node-c288(w182) -> (w184:T20)  [unwired: 3 in]
      n622 = timed-loop {
        timing: w184 -> [_]
        timing-out: [_] -> w183
        stop <- w785 stop-if-true
        n623 = node-c288() -> (w787:bool, w786:i64, w771:i64)  [unwired: 1 in]
        n624 = call-poly <vilib>:"DAQmx Read.vi"("task/channels in"=refnum<k21> "PositionInA") -> ("data"=w753:dbl)  [unwired: 12 in, 2 out]
        n625 = call-poly <vilib>:"DAQmx Read.vi"("task/channels in"=refnum<k21> "PositionInB") -> ("data"=w755:dbl)  [unwired: 12 in, 2 out]
        n626 = call-poly <vilib>:"DAQmx Read.vi"("task/channels in"=refnum<k21> "PositionInC") -> ("data"=w754:dbl)  [unwired: 12 in, 2 out]
        n627 = local write "PIDLoopTime(us)"(w786) -> ()
        n628 = To Double Precision Float(number=w771) -> (double precision float=w770:dbl)
        n629 = local write "PIDSlowLoop"(w787) -> ()
        n630 = expression code="x*1e-6"(w770) -> (w778:dbl)
        n631 = Build Array(w753, w755, w754) -> (w750:dbl[])
        n632 = local write "PIDLoopPeriod(s)"(w778) -> ()
        n633 = Array To Cluster(array=w750) -> (cluster=w760:cluster{"[0]":dbl, "[1]":dbl, "[2]":dbl})
        n634 = local read "BndrsCluster"() -> (w768:T10)
        n635 = local read "PIDGains"() -> (w765:T11)
        n636 = local read "SetPoint"() -> (w769:dbl[])
        n637 = local read "EncMax"() -> (w762:dbl[])
        n638 = local write "EncPos"(w760) -> ()
        n639 = local read "InitialPos"() -> (w729:dbl[])
        n640 = call "PIDBoundaries.vi"("SetPointIn"=w769, "EncPosIn"=w750, "BndrsCluster"=w768, "PIDGainsIn"=w765, "EncMax"=w762) -> ("SetPointOut"=w737:dbl[], "PIDGainsOut"=w761:T12)
        n641 = local read "EncMax"() -> (w730:dbl[])
        n642 = local read "EncPos"() -> (w739:cluster{"[0]":dbl, "[1]":dbl, "[2]":dbl})
        n643 = Array To Cluster(array=w737) -> (cluster=w759:T25)
        n644 = local read "LP_LoadCell(Hz)"() -> (w781:dbl)
        n645 = local read "PIDLoopFreq(Hz)"() -> (w776:dbl)
        n646 = local write "PIDGainsOut"(w761) -> ()
        n647 = Multiply(x=w729, y=w730) -> (x*y=w728:dbl[])
        n648 = local write "SetPtOut"(w759) -> ()
        n649 = feedback #2() -> (w777:dbl)  [unwired: 1 in]
        n650 = feedback-in #2(w776) -> ()
        n651 = feedback #3() -> (w740:dbl)  [unwired: 1 in]
        n652 = feedback-in #3(w781) -> ()
        n653 = Cluster To Array(cluster=w739) -> (array=w736:dbl[])
        n654 = Not Equal?(x=w776, y=w777) -> (x != y?=w774:bool)
        n655 = Subtract(x=w736, y=w728) -> (x-y=w735:dbl[])
        n656 = Not Equal?(x=w781, y=w740) -> (x != y?=w775:bool)
        n657 = Build Array(w775, w774) -> (w773:bool[])
        n658 = Or Array Elements(Boolean array=w773) -> (logical OR=w772:bool)
        n659 = Array Subset(array=w735, index=0, length=2) -> (w738:dbl[])
        n660 = case shown="True" w772 {
          tunnel: [w808 w809] -> w756
          frame False {
            n661 = local read "LP_LoadCell"() -> (w808:T4)
          }
          frame True {
            n662 = local read "LP_LoadCell(Hz)"() -> (w810:dbl)
            n663 = local read "PIDLoopFreq(Hz)"() -> (w811:dbl)
            n664 = call <vilib>:"DFD Butterworth Design.vi"("fs [Hz]"=w811, "filter type"=T23."Lowpass", "low cutoff freq [Hz]"=w810) -> ("filter out"=w809:T4)  [unwired: 7 in, 1 out]
            "LP_LoadCell" <- w809
          }
        }
        n665 = call-poly <vilib>:"DAQmx Write.vi"("task/channels in"=refnum<k21> "PosOutIM", "data"=w738) -> ()  [unwired: 11 in, 3 out]
        n666 = call-poly <vilib>:"DAQmx Read.vi"("task/channels in"=refnum<k21> "ForceInABC") -> ("data"=w727:dbl[])  [unwired: 12 in, 2 out]
        n667 = local read "InitialPos"() -> (w732:dbl[])
        n668 = local read "EncMax"() -> (w731:dbl[])
        n669 = local read "EncPos"() -> (w743:cluster{"[0]":dbl, "[1]":dbl, "[2]":dbl})
        n670 = Multiply(x=w732, y=w731) -> (x*y=w733:dbl[])
        n671 = Cluster To Array(cluster=w743) -> (array=w734:dbl[])
        n672 = Subtract(x=w734, y=w733) -> (x-y=w726:dbl[])
        n673 = call-poly <vilib>:"DFD Filtering.vi"("filter"=w756, "signal in"=w727) -> ("signal out"=w749:dbl[])  [unwired: 2 in, 7 out]
        n674 = Array To Cluster(array=w749) -> (cluster=w758:T26)
        n675 = Index Array(array=w726, index=2) -> (element=w741:dbl)
        n676 = local write "LoadCell"(w758) -> ()
        n677 = call-poly <vilib>:"DAQmx Write.vi"("task/channels in"=refnum<k21> "PosOutT", "data"=w741) -> ()  [unwired: 11 in, 3 out]
        n678 = Negate(x=w726) -> (-x=w724:dbl[])
        n679 = call "PIDDirection.vi"("LoadCellIn"=w749, "SetPointIn"=w737) -> ("MotorDirOut"=w746:bool[])
        n680 = local read "PIDLoopPeriod(s)"() -> (w783:dbl)
        n681 = Negate(x="PIDLimit") -> (-x=w799:dbl)
        n682 = Negate(x="PIDLimit") -> (-x=w796:dbl)
        n683 = Negate(x="PIDLimit") -> (-x=w795:dbl)
        n684 = local read "Linearity"() -> (w764:dbl)
        n685 = Bundle("PIDLimit"="PIDLimit", w799) -> (w794:cluster{"PIDLimit":dbl, dbl})  [unwired: 1 in]
        n686 = Bundle("PIDLimit"="PIDLimit", w796) -> (w793:cluster{"PIDLimit":dbl, dbl})  [unwired: 1 in]
        n687 = Bundle("PIDLimit"="PIDLimit", w795) -> (w792:cluster{"PIDLimit":dbl, dbl})  [unwired: 1 in]
        n688 = Array To Cluster(array=w724) -> (cluster=→"Position, cm":T1)
        n689 = Build Array(w764, w764, w764) -> (w763:dbl[])
        n690 = Build Array(w794, w793, w792) -> (w784:cluster{"PIDLimit":dbl, dbl}[])
        n691 = call-poly <vilib>:"DAQmx Write.vi"("task/channels in"=refnum<k21> "MotorDirABC", "data"=w746) -> ()  [unwired: 11 in, 3 out]
        n692 = call-poly <vilib>:"PID Advanced.vi"("setpoint"=w737, "output range"=w784, "process variable"=w749, "PID gains"=w761, "dt (s)"=w783, "linearity"=w763) -> ("output"=w757:dbl[])  [unwired: 8 in, 1 out]
        n693 = Absolute Value(x=w757) -> (abs(x)=w782:dbl[])
        n694 = Subtract(x=1.0 ("y"), y=w782) -> (x-y=w805:dbl[])
        n695 = local read "PWMFreq(Hz)"() -> (w748:dbl)
        n696 = In Range and Coerce(upper limit=0.999, x=w805, lower limit=0.001) -> (coerced(x)=w790:dbl[])  [unwired: 1 out]
        n697 = local read "PIDLoopFreq(Hz)"() -> (w767:dbl)
        n698 = Index Array(array=w790) -> (element #1=w747:dbl, element #2=w789:dbl, element #3=w788:dbl)  [unwired: 3 in]
        n699 = local read "PWMTaskC"() -> (w779:refnum<k21>)
        n700 = local read "PWMTaskB"() -> (w798:refnum<k21>)
        n701 = local read "PWMTaskA"() -> (w800:refnum<k21>)
        n702 = expression code="(1/x)*1e6"(w767) -> (w766:dbl)
        n703 = call-poly <vilib>:"DAQmx Write.vi"("task/channels in"=w798, "frequency"=w748, "duty cycle"=w789) -> ()  [unwired: 10 in, 3 out]
        n704 = call-poly <vilib>:"DAQmx Write.vi"("task/channels in"=w779, "frequency"=w748, "duty cycle"=w788) -> ()  [unwired: 10 in, 3 out]
        n705 = local read "Stop"() -> (w785:bool)
        n706 = call-poly <vilib>:"DAQmx Write.vi"("task/channels in"=w800, "frequency"=w748, "duty cycle"=w747) -> ()  [unwired: 10 in, 3 out]
        n707 = node-c288(w766) -> ()  [unwired: 1 out]
      }
      n708 = node-c288(w183) -> ()  [unwired: 1 out]
      n709 = node-c288(w180) -> ()  [unwired: 1 out]
    }
    frame #3 {
      n710 = local read "PWMTaskA"() -> (w840:refnum<k21>)
      n711 = local read "PWMTaskB"() -> (w838:refnum<k21>)
      n712 = local read "PWMTaskC"() -> (w832:refnum<k21>)
      n713 = call <vilib>:"DAQmx Stop Task.vi"("task/channels in"=refnum<k21> "sound") -> ("error out"=w827:errorcluster)  [unwired: 13 in, 1 out]
      n714 = call <vilib>:"DAQmx Stop Task.vi"("task/channels in"=refnum<k21> "ForceInABC") -> ("error out"=w843:errorcluster)  [unwired: 13 in, 1 out]
      n715 = call <vilib>:"DAQmx Stop Task.vi"("task/channels in"=refnum<k21> "MotorDirABC") -> ("error out"=w844:errorcluster)  [unwired: 13 in, 1 out]
      n716 = call <vilib>:"DAQmx Clear Task.vi"("task in"=w840) -> ("error out"=w845:errorcluster)  [unwired: 14 in]
      n717 = call <vilib>:"DAQmx Clear Task.vi"("task in"=w838) -> ("error out"=w837:errorcluster)  [unwired: 14 in]
      n718 = call <vilib>:"DAQmx Clear Task.vi"("task in"=w832) -> ("error out"=w833:errorcluster)  [unwired: 14 in]
      n719 = call <vilib>:"DAQmx Stop Task.vi"("task/channels in"=refnum<k21> "PositionInA") -> ("error out"=w846:errorcluster)  [unwired: 13 in, 1 out]
      n720 = call <vilib>:"DAQmx Stop Task.vi"("task/channels in"=refnum<k21> "PositionInB") -> ("error out"=w835:errorcluster)  [unwired: 13 in, 1 out]
      n721 = call <vilib>:"DAQmx Stop Task.vi"("task/channels in"=refnum<k21> "PositionInC") -> ("error out"=w831:errorcluster)  [unwired: 13 in, 1 out]
      n722 = call <vilib>:"DAQmx Stop Task.vi"("task/channels in"=refnum<k21> "PosOutT" ("task")) -> ("error out"=w828:errorcluster)  [unwired: 13 in, 1 out]
      n723 = call <vilib>:"DAQmx Stop Task.vi"("task/channels in"=refnum<k21> "PosOutIM") -> ("error out"=w829:errorcluster)  [unwired: 13 in, 1 out]
      n724 = local write "Stop"(FALSE ("stop")) -> ()
      n725 = call <vilib>:"General Error Handler.vi"("error in (no error)"=w827) -> ()  [unwired: 10 in, 5 out]
      n726 = call <vilib>:"General Error Handler.vi"("error in (no error)"=w843) -> ()  [unwired: 10 in, 5 out]
      n727 = call <vilib>:"General Error Handler.vi"("error in (no error)"=w844) -> ()  [unwired: 10 in, 5 out]
      n728 = call <vilib>:"General Error Handler.vi"("error in (no error)"=w845) -> ()  [unwired: 10 in, 5 out]
      n729 = call <vilib>:"General Error Handler.vi"("error in (no error)"=w837) -> ()  [unwired: 10 in, 5 out]
      n730 = call <vilib>:"General Error Handler.vi"("error in (no error)"=w833) -> ()  [unwired: 10 in, 5 out]
      n731 = call <vilib>:"General Error Handler.vi"("error in (no error)"=w846) -> ()  [unwired: 10 in, 5 out]
      n732 = call <vilib>:"General Error Handler.vi"("error in (no error)"=w835) -> ()  [unwired: 10 in, 5 out]
      n733 = call <vilib>:"General Error Handler.vi"("error in (no error)"=w831) -> ()  [unwired: 10 in, 5 out]
      n734 = call <vilib>:"General Error Handler.vi"("error in (no error)"=w828) -> ()  [unwired: 10 in, 5 out]
      n735 = call <vilib>:"General Error Handler.vi"("error in (no error)"=w829) -> ()  [unwired: 10 in, 5 out]
      n736 = stacked-sequence {
        frame #0 {
          n737 = local read "CerebusFolder"() -> (w855:string)
          n738 = local read "StartTime"() -> (w853:timestamp)
          n739 = local read "TaskType"() -> (w857:string)
          n740 = local read "Monkey"() -> (w852:string)
          n741 = local read "Database"() -> (w858:T14)
          n742 = Empty String/Path?(string/path=w855) -> (empty?=w856:bool)
          n743 = Bundle By Name(cluster=w858, "NHPName"=w852, "ExperimentDate"=w853, "CerebusFolder"=w855, "TaskType"=w857) -> (w851:T14)
          n744 = case shown="False" w856 {
            frame False {
            }
            frame True {
              n745 = One Button Dialog(message="The Cerebus data folder is unknown\nand will not be saved to the database.\nMake sure to update the database\nmanually with the appropriate folder\nname!") -> ()  [unwired: 1 in, 1 out]
            }
          }
          n746 = local write "Database"(w851) -> ()
          n747 = call "SendDatabase2Cerebus.vi"("Database"=w851) -> ("ParameterString"=w847:string)
          n748 = call "UpdateDatabaseRemote.vi"("Database"=w851, "CallType"=enum16{"Initialize", "Save", "Load"}."Save") -> ()  [unwired: 1 in, 3 out]
          n749 = Concatenate Strings("TaskParameters:" ("string"), w847) -> (w848:string)
          n750 = call "SendCerebus8.vi"("String"=w848, "Mode"=T16."String") -> ()  [unwired: 3 in]
        }
        frame #1 {
          # "Stop Cerebus recording"
          n751 = local read "StopRecording"() -> (w860:bool)
          n752 = case shown="True" w860 {
            frame False {
            }
            frame True {
              n753 = local read "AutoCentraVI"() -> (w862:path)
              n754 = Open Application Reference(10:u16 3362 ("port number or service name (3363)"), 11:"192.168.0.1" ("machine name (\"\":  open local reference)")) -> (0:w865:errorcluster, 3:w867:refnum<vi>)  [unwired: 2 in]
              n755 = Open VI Reference(type specifier VI Refnum (for type only)=refnum<vi> refnum, application reference (local)=w867, vi path=w862, error in (no error)=w865) -> (vi reference=w863:refnum<vi>, error out=w864:errorcluster)  [unwired: 2 in]
              n756 = call-by-ref "?"(reference=w863, error in=w864, "Mode"=T19."StopRecording") -> ("Recording?"=w861:bool)  [unwired: 2 in, 4 out]
              n757 = local write "Recording?"(w861) -> ()
            }
          }
        }
        frame #2 {
          n758 = property class="App"() -> ("Disp.AllMonitors"=w878:T27)  [unwired: 2 in, 2 out]
          n759 = Array To Cluster(array=w878) -> (cluster=w877:T28)
          n760 = Unbundle By Name(w877) -> ("Disp.AllMonitors[0].Bounds.Right"=w873:i16, "Disp.AllMonitors[0].Bounds.Bottom"=w872:i16)
          n761 = property class="VI"() -> ("Front Panel.WinBounds"=w876:T29)  [unwired: 2 in, 2 out]
          n762 = Bundle By Name(cluster=w876, "Left"=i16 65 ("left"), "Top"=i16 0 ("top"), "Right"=w873, "Bottom"=w872) -> (w871:T29)
          n763 = property class="VI"("Front Panel.WinBounds"=w871) -> ()  [unwired: 2 in, 2 out]
        }
        frame #3 {
          n764 = call "SendCerebus32.vi"("Mode"=T16."Close") -> ()  [unwired: 4 in]
        }
      }
    }
  }
